vi "State Machine from Enum.vi"(6 "Variant in":variant, 7 "Shift Pressed?":bool, 8 "error in (no error)":errorcluster, 10 "QD Combo Box Ref":refnum<vi>, 11 "QD Launch VI Ref":refnum<vi>) -> (0 "error out":errorcluster, 4 "Variant out":variant)   [LabVIEW 2012, in "State Machine From Enum.lvlib"]
doc: "Goal :\n\nPretty much everyone uses state machines as this is a rather basic but efficient design pattern that can be mixed together with others DPs. Whichever the platform (RT, FPGA, Win), an application will most likely include a state machine (or more!).\n\nFirst thing : create the enum that will describe the states of the machine. Yeah well, with this QDKS, that's roughly the only thing you will need to do.\n\nHow-To :\n\n- Copy the attached QD VI to the usual directory.\n\n- Configure its key (S is fine !)\n\n- Select an enum terminal or constant in your BD. Make sure there is some free space at the right of the enum.\n\n- Ctrl+Space Ctrl+Key. You've earned a state machine corresponding to the enum items.\n\nDefault Shortcut - [S]"
uses:
  State Machine From Enum.lvlib
  <vilib>/Utility/miscctls.llb/LVPointTypeDef.ctl
  <vilib>/Utility/miscctls.llb/LVBoundsTypeDef.ctl
  <vilib>/Utility/miscctls.llb/LVPositionTypeDef.ctl
panel:
  in  "Undo Name":string="Quick Drop Keyboard Shortcut"
  # "Do not change the connector pane of this VI.\n\nSee the block diagram for directions on how to use this template."
  # "Specify the name of the Undo transaction"
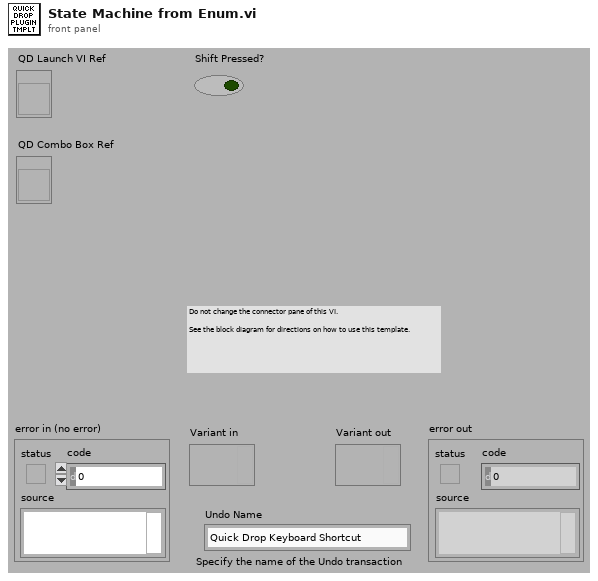
[diagram p1: front panel]
types:
  T1 = typedef "LVPositionTypeDef.ctl" = cluster{"Left":i32, "Top":i32}
  T2 = typedef "LVBoundsTypeDef.ctl" = cluster{"Width":u32, "Height":u32}
  T3 = typedef "LVPointTypeDef.ctl" = cluster{"Horizontal":i16, "Vertical":i16}
  T4 = enum32{"not a typedef", "typedef", "strict typedef", "class private data"}
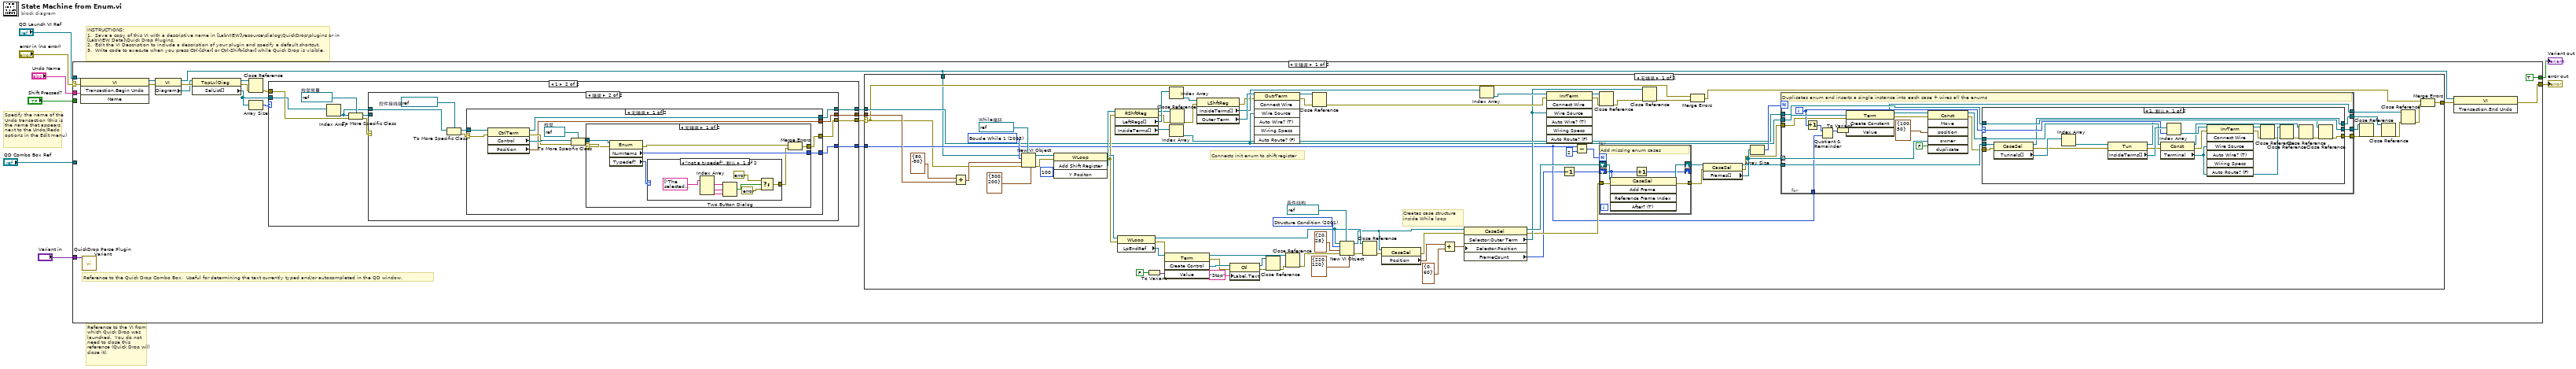
[diagram p0: block diagram]
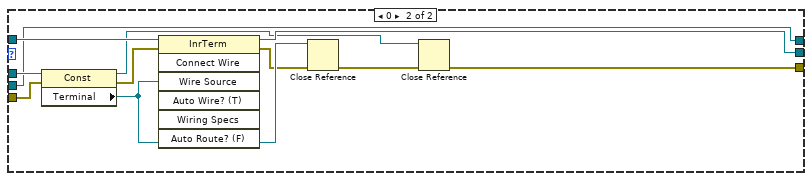
[diagram p2: hidden frame]
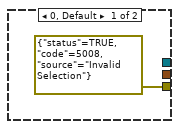
[diagram p4: hidden frame]
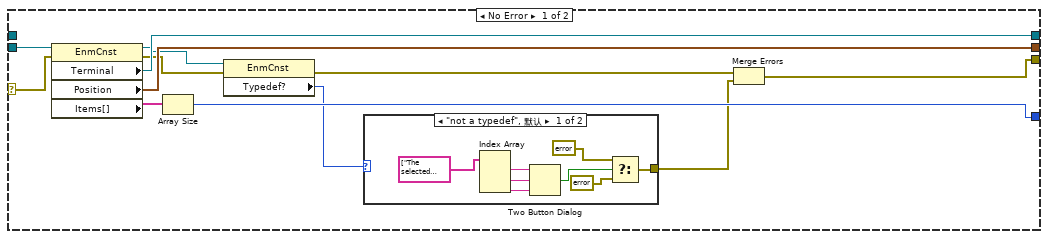
[diagram p5: hidden frame]
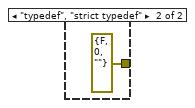
[diagram p6: hidden frame]
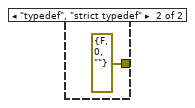
[diagram p7: hidden frame]
diagram:
  # "Specify the name of the Undo transaction (this is the name that appears next to the Undo/Redo options in the Edit menu)"
  # "Reference to the VI from which Quick Drop was launched.  You do not need to close this reference (Quick Drop will close it)."
  # "INSTRUCTIONS:\n1.  Save a copy of this VI with a descriptive name in [LabVIEW]\\resource\\dialog\\QuickDrop\\plugins or in [LabVIEW Data]\\Quick Drop Plugins.\n2.  Edit the VI Description to include a description of your plugin and specify a default shortcut. \n3.  Write code to execute when you press Ctrl-[char] or Ctrl-Shift-[char] while Quick Drop is visible."
  n1 = case shown="无错误" "error in (no error)" {
    selector: "error in (no error)" -> [w28 w239]
    tunnel: [w23 w239] -> w7
    tunnel: "QD Launch VI Ref" -> [w27 _]
    tunnel: "Shift Pressed?" -> [_ _]
    tunnel: "QD Combo Box Ref" -> [_ _]
    tunnel: "Variant in" -> [w29 _]
    tunnel: "Undo Name" -> [w26 _]
    tunnel: [TRUE _] -> w1
    frame No Error {
      # "Reference to the Quick Drop Combo Box.  Useful for determining the text currently typed and/or autocompleted in the QD window."
      n2 = invoke class="VI" method="Transaction.Begin Undo"(reference=w27, error in=w28, "Name"=w26) -> (reference out=w22:refnum<vi>, error out=w24:errorcluster)  [unwired: 1 in, 2 out]
      n3 = call <vilib>:"QuickDrop Parse Plugin Variant.vi"("QDKS Variant in"=w29) -> ()  [unwired: 12 in, 3 out]
      n4 = property class="VI"(reference=w22, error in=w24) -> (reference out=w9:refnum<vi>, error out=w17:errorcluster, "Diagram"=w16:refnum<vi>)
      n5 = property class="TopLvlDiag"(reference=w16, error in=w17) -> (reference out=w14:refnum<vi>, error out=w15:errorcluster, "SelList[]"=w20:refnum<vi>[])
      n6 = Close Reference(reference=w14, error in (no error)=w15) -> (error out=w19:errorcluster)
      n7 = Array Size(array=w20) -> (size(s)=w21:i32)
      n8 = case shown="1" w21 {
        tunnel: w20 -> [_ w180]
        tunnel: w19 -> [_ w179]
        tunnel: [errorcluster {"status"=TRUE, "code"=5008, "source"="Invalid Selection"} ("error IO") w178] -> w18
        tunnel: [_ w174] -> w12
        tunnel: [_ w173] -> w11
        tunnel: [_ w172] -> w10
        frame 0, Default {
        }
        frame 1 {
          w176 = refnum<vi> refnum  # 枚举常量
          n9 = Index Array(array=w180) -> (element=w171:refnum<vi>)  [unwired: 1 in]
          n10 = To More Specific Class(target class=w176, reference=w171, error in=w179) -> (specific class reference=w177:refnum<vi>, error out=w175:errorcluster)
          n11 = case shown="错误" w175 {
            selector: w175 -> [w190 _]
            tunnel: [w183 w206] -> w178
            tunnel: w177 -> [w191 _]
            tunnel: [w189 w205] -> w172
            tunnel: [w188 w204] -> w174
            tunnel: [w187 w203] -> w173
            tunnel: w171 -> [_ w202]
            frame No Error {
              n12 = property class="EnmCnst"(reference=w191, error in=w190) -> (reference out=w186:refnum<vi>, error out=w184:errorcluster, "Terminal"=w189:refnum<vi>, "Position"=w188:T1, "Items[]"=w192:string[])
              n13 = Array Size(array=w192) -> (size(s)=w187:i32)
              n14 = property class="EnmCnst"(reference=w186, error in=w184) -> (error out=w181:errorcluster, "Typedef?"=w185:T4)  [unwired: 1 out]
              n15 = case shown="\"not a typedef\", 默认" w185 {
                tunnel: [w193 errorcluster {"status"=FALSE, "code"=0, "source"=""} ("error IO")] -> w182
                frame "not a typedef", Default {
                  n16 = Index Array(array=string[] ["The selected enum is not a typedef (and you may not create a non-typedef'ed state machine !). \n\nDo you want to continue ?", "Yes", "No"]) -> (element #1=w199:string, element #2=w198:string, element #3=w197:string)  [unwired: 3 in]
                  n17 = Two Button Dialog(message=w199, 1:w197, 2:w198) -> (T button?=w196:bool)
                  n18 = Select(t=errorcluster {"status"=FALSE, "code"=0, "source"=" "} ("error IO"), s=w196, f=errorcluster {"status"=TRUE, "code"=5008, "source"="Invalid Selection"} ("error IO")) -> (s? t:f=w193:errorcluster)
                }
                frame "typedef", "strict typedef" {
                }
              }
              n19 = Merge Errors(w181, w182) -> (w183:errorcluster)
            }
            frame Error {
              w208 = refnum<vi> refnum  # 控件接线端
              n20 = To More Specific Class(target class=w208, reference=w202) -> (specific class reference=w209:refnum<vi>, error out=w207:errorcluster)  [unwired: 1 in]
              n21 = case shown="无错误" w207 {
                selector: w207 -> [w214 w238]
                tunnel: w209 -> [w220 _]
                tunnel: [w213 w238] -> w206
                tunnel: [w212 _] -> w205
                tunnel: [w211 _] -> w204
                tunnel: [w210 _] -> w203
                frame No Error {
                  w217 = refnum<vi> refnum  # 枚举
                  n22 = property class="CtrlTerm"(reference=w220, error in=w214) -> (reference out=w212:refnum<vi>, error out=w218:errorcluster, "Control"=w219:refnum<vi>, "Position"=w211:T1)
                  n23 = To More Specific Class(target class=w217, reference=w219, error in=w218) -> (specific class reference=w216:refnum<vi>, error out=w215:errorcluster)
                  n24 = case shown="无错误" w215 {
                    selector: w215 -> [w226 w237]
                    tunnel: w216 -> [w227 _]
                    tunnel: [w221 w237] -> w213
                    tunnel: [w225 _] -> w210
                    frame No Error {
                      n25 = property class="Enum"(reference=w227, error in=w226) -> (error out=w222:errorcluster, "NumItems"=w225:u32, "Typedef?"=w224:T4)  [unwired: 1 out]
                      n26 = case shown="\"not a typedef\", 默认" w224 {
                        tunnel: [w228 errorcluster {"status"=FALSE, "code"=0, "source"=""} ("error IO")] -> w223
                        frame "not a typedef", Default {
                          n27 = Index Array(array=string[] ["The selected enum is not a typedef (and you may not create a non-typedef'ed state machine !). \n\nDo you want to continue ?", "Yes", "No"]) -> (element #1=w234:string, element #2=w233:string, element #3=w232:string)  [unwired: 3 in]
                          n28 = Two Button Dialog(message=w234, 1:w232, 2:w233) -> (T button?=w231:bool)
                          n29 = Select(t=errorcluster {"status"=FALSE, "code"=0, "source"=" "} ("error IO"), s=w231, f=errorcluster {"status"=TRUE, "code"=5008, "source"="Invalid Selection"} ("error IO")) -> (s? t:f=w228:errorcluster)
                        }
                        frame "typedef", "strict typedef" {
                        }
                      }
                      n30 = Merge Errors(w222, w223) -> (w221:errorcluster)
                    }
                    frame Error {
                    }
                  }
                }
                frame Error {
                }
              }
            }
          }
        }
      }
      n31 = case shown="无错误" w18 {
        selector: w18 -> [w46 w169]
        tunnel: [w44 w169] -> w13
        tunnel: w12 -> [w49 _]
        tunnel: w11 -> [w48 _]
        tunnel: w10 -> [w47 _]
        tunnel: w9 -> [w45 _]
        frame No Error {
          w98 = refnum<vi> refnum  # 条件结构
          w99 = 2001 items=[" Additionner (avec terminaux d'erreur)"=3915, " Arbre (classique)"=21819, " Arbre (moderne)"=21793, " Arbre (système)"=21794, " Barre de défil. horiz. de dlg"=21905, " Barre de défil. vert. de dlg"=21906, " Barre de progression horizontale (moderne)"=21102, " Barre de progression horizontale (système)"=21910, " Barre de progression verticale (moderne)"=21104, " Barre de progression verticale (système)"=21909, " Bin 1"=3073, " Bin 2"=21755, " Boucle While 1"=2003, " Boucle While 2"=2352, " Bouton Annuler (moderne)"=21739, " Bouton Annuler (système)"=3131, " Bouton OK (moderne)"=21738, " Bouton OK (système)"=3130, " Bouton radio (système)"=3133, " Bouton rotatif (classique)"=3005, " Bouton rotatif (moderne)"=21000, " Bouton-poussoir carré"=3119, " Bouton-poussoir carré (profil)"=3113, " Bouton-poussoir circulaire"=3118, " Bouton-poussoir circulaire (profil)"=3112, " Boutons radio (classique)"=22003, " Boutons radio (moderne)"=22001, " Boutons radio (système)"=22002, " Boîte de couleur encadrée (classique)"=3008, " Boîte de couleur encadrée (moderne)"=21019, " Boîte de dialogue de fichier (obsolète)"=8081, " Boîte en relief (classique)"=3600, " Boîte en relief (moderne)"=3637, " Boîte épaisse (encastrée)"=3635, " Cadran (classique)"=3050, " Cadran (moderne)"=21732, " Cadre encastré (moderne)"=3607, " Cadre encastré (système)"=3624, " Case à cocher (classique)"=3117, " Case à cocher (moderne)"=21924, " Case à cocher (système)"=3132, " Case à cocher mixte (système)"=21333, " Chaîne de dlg"=2110, " Chaîne déroulante (classique)"=3304, " Chaîne déroulante (moderne)"=21604, " Chaîne déroulante (système)"=21917, " Cluster (classique)"=3400, " Cluster (moderne)"=21607, " Commande chaîne (classique)"=3200, " Commande chaîne (moderne)"=21701, " Commande chaîne (système)"=21920, " Commande chemin (classique)"=3203, " Commande chemin (moderne)"=21730, " Commande chemin (système)"=21922, " Commande horodatage (classique)"=5555, " Commande horodatage (moderne)"=21913, " Commande horodatage (système)"=21967, " Commande numérique (classique)"=3000, " Commande numérique (moderne)"=21003, " Commande numérique (système)"=21919, " Commande numérique à incrémentation (système)"=21900, " Commande onglets (classique)"=3330, " Commande onglets (moderne)"=3332, " Commande onglets (système)"=3331, " Commande variable partagée (classique)"=3472, " Commande variable partagée (moderne)"=21814, " Copier (obsolète)"=1416, " Coude gauche vers le bas (ombré)"=3711, " Coude gauche vers le bas (plat)"=3811, " Coude gauche vers le haut (ombré)"=3708, " Coude gauche vers le haut (plat)"=3808, " Coude vers le bas à droite (ombré)"=3717, " Coude vers le bas à droite (plat)"=3817, " Coude vers le haut à droite (ombré)"=3714, " Coude vers le haut à droite (plat)"=3814, " Diviser (avec terminaux d'erreur)"=3918, " Données numériques (classique)"=3210, " Données numériques (moderne)"=21216, " Déplacer (obsolète)"=1415, " Entonnoir 1"=21754, " Entonnoir 2"=3072, " Fermer un fichier (obsolète)"=1405, " Glissière horizontale (classique)"=3010, " Glissière horizontale (système)"=21904, " Glissière verticale (système)"=21903, " Glissière à curseur horizontale (classique)"=3011, " Glissière à curseur horizontale (moderne)"=21101, " Glissière à curseur horizontale (système)"=21902, " Glissière à curseur verticale (classique)"=3007, " Glissière à curseur verticale (moderne)"=21017, " Glissière à curseur verticale (système)"=21901, " Glissière à niveau horizontale (classique)"=3012, " Glissière à niveau horizontale (moderne)"=21100, " Glissière à niveau verticale (classique)"=3009, " Glissière à niveau verticale (moderne)"=21014, " Graphe (classique)"=3504, " Graphe (moderne)"=21703, " Graphe d'intensité (classique)"=3510, " Graphe d'intensité (moderne)"=21720, " Graphe déroulant (moderne)"=21717, " Graphe déroulant d'intensité (classique)"=3509, " Graphe déroulant d'intensité (moderne)"=21719, " Graphe numérique (classique)"=3511, " Graphe numérique (moderne)"=21718, " Graphe XY (classique)"=3500, " Graphe XY (moderne)"=21716, " Horodatage (constante du diagramme)"=2068, " Indicateur chaîne (classique)"=3201, " Indicateur chaîne (moderne)"=21702, " Indicateur chemin (classique)"=3204, " Indicateur chemin (moderne)"=21731, " Indicateur horodatage (classique)"=5556, " Indicateur horodatage (moderne)"=21914, " Indicateur numérique (classique)"=3001, " Indicateur numérique (moderne)"=21004, " Infos sur le fichier/répertoire (obsolète)"=1413, " Interface CAN (classique)"=3339, " Interface CAN (constante du diagramme)"=2123, " Interface CAN (moderne)"=21815, " Interface CAN (système)"=21964, " Interrupteur à bascule horizontal (classique)"=3110, " Interrupteur à bascule horizontal (moderne)"=21700, " Interrupteur à bascule vertical (classique)"=3111, " Interrupteur à bascule vertical (moderne)"=21005, " Interrupteur à glissière vertical (classique)"=3115, " Interrupteur à glissière vertical (moderne)"=21741, " Jauge (classique)"=3040, " Jauge (moderne)"=21009, " LED carrée (classique)"=3121, " LED carrée (moderne)"=21013, " LED circulaire (classique)"=3120, " LED circulaire (moderne)"=21012, " Ligne (ciselée, fine)"=3627, " Ligne (ciselée, système)"=3632, " Ligne (ciselée, épaisse)"=3630, " Ligne (fine)"=3626, " Ligne (épaisse)"=3629, " Ligne avec flèche (fine)"=3628, " Ligne avec flèche (épaisse)"=3631, " Liste déroulante (classique)"=21806, " Liste déroulante (moderne)"=21792, " Liste déroulante (système)"=21805, " Liste multicolonne (classique)"=21799, " Liste multicolonne (moderne)"=21791, " Liste multicolonne (système)"=21798, " Menu déroulant (classique)"=3018, " Menu déroulant (moderne)"=21600, " Menu déroulant d'images (classique)"=3015, " Menu déroulant d'images (moderne)"=21602, " Menu déroulant d'images (système)"=21925, " Menu déroulant texte (classique)"=3014, " Menu déroulant texte (constante du diagramme)"=2008, " Menu déroulant texte (moderne)"=21601, " Menu déroulant texte (système)"=3060, " Menu déroulant texte et images (classique)"=3016, " Menu déroulant texte et images (moderne)"=21603, " Mettre à jour le fichier (obsolète)"=1406, " Moteur (ombré)"=3720, " Moteur (plat)"=3820, " Multiplier (avec terminaux d'erreur)"=3917, " Nom d'échelle DAQmx (classique)"=3317, " Nom d'échelle DAQmx (constante du diagramme)"=2116, " Nom d'échelle DAQmx (moderne)"=21775, " Nom d'échelle DAQmx (système)"=21952, " Nom de périphérique DAQmx (classique)"=3318, " Nom de périphérique DAQmx (constante du diagramme)"=2093, " Nom de périphérique DAQmx (moderne)"=21773, " Nom de périphérique DAQmx (système)"=21950, " Nom de ressource VISA (classique)"=3409, " Nom de ressource VISA (moderne)"=21737, " Nom de tâche DAQmx (classique)"=3442, " Nom de tâche DAQmx (constante du diagramme)"=3434, " Nom de tâche DAQmx (moderne)"=21778, " Nom de tâche DAQmx (système)"=21959, " Nom logique IVI (classique)"=3414, " Nom logique IVI (constante du diagramme)"=3420, " Nom logique IVI (moderne)"=21736, " Numérique de dlg 1"=2100, " Numérique de dlg 2"=3006, " Pixmap (attention : dangereux)"=3507, " Point d'E/S FieldPoint (classique)"=3439, " Point d'E/S FieldPoint (constante du diagramme)"=3440, " Point d'E/S FieldPoint (moderne)"=21784, " Pompe vers la droite (ombrée)"=3719, " Pompe vers la droite (plate)"=3819, " Pompe vers la gauche (ombrée)"=3713, " Pompe vers la gauche (plate)"=3813, " RecomposerRéfValDonnéesDéverrou (warning: dangerous)"=2407, " RecomposerVariant (warning: dangerous)"=2405, " Rectangle de couleur (brisé ?)"=3625, " Ressource Motion (classique)"=3448, " Ressource Motion (constante du diagramme)"=3449, " Ressource Motion (moderne)"=21787, " Réservoir (classique)"=3020, " Réservoir (moderne)"=21006, " Réservoir atmosphérique (classique)"=3070, " Réservoir atmosphérique (moderne)"=21751, " Réservoir de pression (ombré)"=21753, " Réservoir de pression (plat)"=3075, " Réservoir ouvert (ombré classique)"=3074, " Réservoir ouvert (plat classique)"=21752, " Soupape courbée vers la droite (contour)"=3805, " Soupape courbée vers la droite (ombrée)"=21765, " Soupape courbée vers la droite (plate)"=3705, " Soupape courbée vers la gauche (contour)"=3801, " Soupape courbée vers la gauche (ombrée)"=21761, " Soupape courbée vers la gauche (plate)"=3701, " Soupape courbée vers le bas (contour)"=3807, " Soupape courbée vers le bas (ombrée)"=21767, " Soupape courbée vers le bas (plate)"=3707, " Soupape courbée vers le haut (contour)"=3803, " Soupape courbée vers le haut (ombrée)"=21763, " Soupape courbée vers le haut (plate)"=3703, " Soupape rectangulaire vers la droite (contour)"=3804, " Soupape rectangulaire vers la droite (ombrée)"=21764, " Soupape rectangulaire vers la droite (plate)"=3704, " Soupape rectangulaire vers la gauche (contour)"=3800, " Soupape rectangulaire vers la gauche (ombrée)"=21760, " Soupape rectangulaire vers la gauche (plate)"=3700, " Soupape rectangulaire vers le bas (contour)"=3806, " Soupape rectangulaire vers le bas (ombrée)"=21766, " Soupape rectangulaire vers le bas (plate)"=3706, " Soupape rectangulaire vers le haut (contour)"=21762, " Soupape rectangulaire vers le haut (ombrée)"=3802, " Soupape rectangulaire vers le haut (plate)"=3702, " Source de déclenchement analogique DAQmx (classique)"=3336, " Source de déclenchement analogique DAQmx (constante du diagramme)"=2119, " Source de déclenchement analogique DAQmx (moderne)"=21774, " Source de déclenchement analogique DAQmx (système)"=21951, " Soustraire (avec terminaux d'erreur)"=3916, " Supprimer (obsolète)"=1417, " Switch DAQmx (classique)"=3337, " Switch DAQmx (constante du diagramme)"=2121, " Switch DAQmx (moderne)"=21776, " Switch DAQmx (système)"=21953, " Table (classique)"=21796, " Table (moderne)"=21790, " Table (système)"=21797, " Tableau (classique)"=3300, " Tableau (constante du diagramme)"=2070, " Tableau (moderne)"=21608, " Tag de refnum défini par l'utilisateur (classique)"=3429, " Tag de refnum défini par l'utilisateur (constante du diagramme)"=3426, " Tag de refnum défini par l'utilisateur (moderne)"=21745, " Tag de refnum défini par l'utilisateur aplati (classique)"=3454, " Tag de refnum défini par l'utilisateur aplati (modern)"=21747, " Tag défini par l'utilisateur aplati (moderne)"=21749, " Tag défini par utilisateur (classique)"=3329, " Tag défini par utilisateur (constante du diagramme)"=2114, " Tee vers la droite (ombré)"=3715, " Tee vers la droite (plat)"=3815, " Tee vers la gauche (ombré)"=3709, " Tee vers la gauche (plat)"=3809, " Tee vers le bas (ombré)"=3718, " Tee vers le bas (plat)"=3818, " Tee vers le haut (ombré)"=3712, " Tee vers le haut (plat)"=3812, " Terminal DAQmx (classique)"=3319, " Terminal DAQmx (constante du diagramme)"=2117, " Terminal DAQmx (moderne)"=21781, " Terminal DAQmx (système)"=21955, " Thermomètre (classique)"=3021, " Thermomètre (moderne)"=21007, " Tuyau horiz. (ombré)"=3710, " Tuyau horiz. (plat)"=3810, " Tuyau vertical (ombré)"=3716, " Tuyau vertical (plat)"=3816, " Tâche CAN (classique)"=3470, " Tâche CAN (constante du diagramme)"=3471, " Tâche CAN (moderne)"=21789, " Tâche CAN (système)"=21963, " Voie CAN (classique)"=3340, " Voie CAN (constante du diagramme)"=2124, " Voie CAN (moderne)"=21817, " Voie CAN (système)"=21966, " Voie de NI-DAQ traditionnel (classique)"=3320, " Voie de NI-DAQ traditionnel (constante du diagramme)"=2085, " Voie de NI-DAQ traditionnel (moderne)"=21733, " Voie globale DAQmx (classique)"=3443, " Voie globale DAQmx (constante du diagramme)"=3430, " Voie globale DAQmx (moderne)"=21770, " Voie globale DAQmx (système)"=21957, " Voie physique DAQmx (classique)"=3335, " Voie physique DAQmx (constante du diagramme)"=2118, " Voie physique DAQmx (moderne)"=21777, " Voie physique DAQmx (système)"=21954, " Vumètre (classique)"=3030, " Vumètre (moderne)"=21008, " Écrire dans un fichier binaire"=8078, " Écrire dans un fichier texte"=8080, " Énum (classique)"=3023, " Énum (moderne)"=21605, " Énum (système)"=3062, " Étiquette (moderne)"=21960, " Étiquette (système)"=21961, "Activer le repérage des menus"=9002, "Adapter d'entier à virgule fixe"=5567, "Adapter de virgule fixe à entier"=5566, "Adapter le type"=1166, "Additionner"=1050, "Additionner les éléments du tableau"=1903, "Agitateur"=3831, "Ajouter la chaîne Vrai/Faux"=1511, "Ajouter un élément au début d'une file d'attente"=9129, "Ajouter un élément à la fin d'une file d'attente"=9111, "Ajouter un élément à la fin d'une file d'attente avec pertes"=9130, "Ajouter une chaîne multiligne"=1510, "AllSpoll"=1960, "Ampoule carrée"=3105, "Ampoule circulaire"=3104, "Ancien VISA Open"=1921, "Annuler une notification"=9107, "Aperçu du premier élément d'une file d'attente"=9112, "Aplatir en chaîne"=1164, "Aplatir en XML"=8400, "Appel par référence MathScript"=3906, "Appeler la méthode parente"=2354, "Appeler par référence"=3901, "Appeler une fonction d'une DLL"=2062, "Arc cosinus"=1207, "Arc cosinus hyperbolique"=1218, "Arc cosécante"=23050, "Arc cosécante hyperbolique"=23056, "Arc cotangente"=23052, "Arc cotangente hyperbolique"=23058, "Arc sinus"=1206, "Arc sinus hyperbolique"=1217, "Arc sécante"=23051, "Arc sécante hyperbolique"=23057, "Arc tangente"=1208, "Arc tangente (2 entrées)"=1228, "Arc tangente hyperbolique"=1219, "Array Interface Control"=23777, "Arrondir vers +l'infini"=1076, "Arrondir vers -l'infini"=1075, "Arrondir à l'entier le plus proche"=1055, "Arrêter"=1350, "Assembler"=2049, "Assembler des signaux"=2350, "Assembler par nom"=2057, "Attendre (ms)"=1302, "Attendre un multiple de ms"=1327, "Attendre une activité sur la face-avant"=1328, "Attendre une notification"=9105, "Attendre une notification avec historique des notificateurs"=9131, "Attendre une notification de plusieurs"=9106, "Attendre une notification de plusieurs avec historique des notificateurs"=9132, "Attendre une occurrence"=1701, "Attente d'activité"=1722, "Automation Fermer"=8001, "Automation Ouvrir"=8000, "Balayer un fichier"=2082, "Balayer une chaîne"=2080, "Balayer une valeur"=1534, "Barre de division horizontale"=21861, "Barre de division horizontale (classique)"=21863, "Barre de division horizontale (système)"=21865, "Barre de division verticale"=21860, "Barre de division verticale (classique)"=21862, "Barre de division verticale (système)"=21864, "Barre de défilement horizontale"=21110, "Barre de défilement verticale"=21111, "Barre de menus du VI actuel"=9000, "Barre graduée horizontale"=21106, "Barre graduée verticale"=21107, "Base du logarithme népérien"=23510, "Bibliothèque de VIs"=1425, "Bitpack en tableau"=3135, "Bluetooth - Attendre un récepteur"=9147, "Bluetooth - Créer un récepteur"=9151, "Bluetooth - Découvrir"=9152, "Bluetooth - Fermer la connexion"=9148, "Bluetooth - Lire"=9149, "Bluetooth - Ouvrir une connexion"=9153, "Bluetooth - Écrire"=9150, "Booléen en (0,1)"=1167, "Boucle cadencée"=5570, "Boucle de contrôle et simulation"=2099, "Boucle For"=2002, "Bouton allongé à étiquette"=3125, "Bouton carré"=3101, "Bouton carré plat"=3103, "Bouton carré plat de plate-forme"=3134, "Bouton carré à étiquette"=3123, "Bouton circulaire"=3100, "Bouton circulaire à étiquette"=3122, "Bouton LED"=3116, "Bouton radio carré"=3107, "Bouton radio circulaire"=3106, "Bouton rectangulaire à étiquette"=3124, "Bouton rond plat"=3102, "Bouton Stop"=21230, "Bouton Stop circulaire"=3127, "Bouton Stop rectangulaire"=3128, "Bouton Texte"=21015, "Bouton-poussoir"=21001, "Boîte arrondie en relief"=3609, "Boîte arrondie encastrée"=3638, "Boîte arrondie encastrée 1"=3610, "Boîte arrondie plate"=3611, "Boîte bouton horizontale"=3636, "Boîte de calcul"=2004, "Boîte de couleur"=3013, "Boîte de couleur à bord mince"=2905, "Boîte de dialogue de fichier"=8058, "Boîte de dialogue à deux boutons"=1341, "Boîte de dialogue à un bouton"=1340, "Boîte encastrée"=3601, "Boîte lisse horizontale"=3633, "Boîte lisse verticale"=3634, "Boîte plate"=3602, "Cadre en relief"=3606, "Cadre plat"=3608, "Carré"=23059, "Casting dynamique d'interface FPGA"=5690, "Cercle en relief"=3603, "Cercle encastré"=3604, "Cercle plat"=3605, "Changer les bases d'unités"=1079, "Charge élémentaire (C)"=23517, "Chaîne aplatie en variant"=8202, "Chaîne au format tableur en tableau"=1539, "Chaîne d'appel"=1999, "Chaîne de date/heure"=1600, "Chaîne décimale en nombre"=1184, "Chaîne en chemin"=1078, "Chaîne en IP"=1711, "Chaîne en tableau d'octets"=1608, "Chaîne en variable partagée"=1830, "Chaîne Fract/Exp en nombre"=1187, "Chaîne hexadécimale en nombre"=1185, "Chaîne octale en nombre"=1186, "Chaîne simple"=2115, "Chemin du VI actuel"=1426, "Chemin en chaîne"=1077, "Chemin en tableau de chaînes"=1423, "Chemin/Chaîne vide ?"=1112, "Chiffre décimal ?"=1119, "Chiffre hexa ?"=1123, "Chiffre octal ?"=1129, "Classe lexicale"=1126, "Classer un tableau 1D"=1120, "Cluster en tableau"=1169, "Code Interface Node"=2050, "Commande Plug-In"=21820, "Commande/état du périphérique"=1433, "Complexe conjugué"=1048, "Complexe en polaire"=1045, "Complexe en Réel/Im"=1044, "Composer un chemin"=1419, "Compresseur"=3832, "Compteur d'impulsions d'horloge (ms)"=1300, "Concaténer des chaînes"=2040, "Constante 'Pas un chemin'"=23524, "Constante 'Pas un refnum'"=23526, "Constante boîte de couleur"=2120, "Constante chaîne"=2007, "Constante chaîne déroulante"=2088, "Constante chaîne vide"=23503, "Constante chemin"=2009, "Constante chemin vide"=23523, "Constante cluster"=2071, "Constante d'Avogadro (1/mol)"=23520, "Constante de Planck (J/Hz)"=23516, "Constante de Rydberg (1/m)"=23521, "Constante de spécification de classe"=2094, "Constante de spécification de classe de variable"=2106, "Constante des gaz parfaits (J/(mol K))"=23522, "Constante Faux"=2006, "Constante fin de ligne"=23525, "Constante gravitationnelle"=23519, "Constante menu déroulant d'erreurs"=2039, "Constante menu déroulant de symboles"=2038, "Constante Nom de variable"=3478, "Constante numérique"=2005, "Constante Retour chariot"=23500, "Constante Retour à la ligne"=23501, "Constante référence de valeur de données"=24134, "Constante tabulation"=23502, "Constante variable partagée"=3473, "Constante énumération"=2090, "Construire un tableau"=2041, "Construire un tableau de clusters"=2047, "Construire une matrice"=8500, "Construire une waveform"=2066, "Conteneur .NET"=2125, "Conteneur ActiveX"=2072, "Contraindre au type"=2402, "Contrôle de l'aide en ligne"=1355, "Contrôle de la fenêtre d'aide"=1353, "Convertir une unité"=2059, "Copier"=8053, "Correspondance de chaîne Vrai/Faux"=1533, "Cosinus"=1201, "Cosinus hyperbolique"=1215, "Cosécante"=1204, "Cosécante hyperbolique"=23053, "Cotangente"=1205, "Cotangente hyperbolique"=23055, "Créer l'extrémité d'écriture d'un flux réseau"=23810, "Créer l'extrémité de lecture d'un flux réseau"=23811, "Créer un dossier"=8055, "Créer un flux"=23796, "Créer un événement utilisateur"=2073, "Créer une FIFO RT"=24000, "Culbuteur"=21002, "Culbuteur vertical"=21740, "Dans la gamme"=1127, "DataSocket Fermer"=1085, "DataSocket Lire"=1086, "DataSocket Ouvrir"=1084, "DataSocket Écrire"=1087, "Date et heure en secondes"=1303, "Date/heure en secondes"=1308, "Demander une désallocation"=1610, "DevClear"=1961, "DevClearList"=1962, "Diagramme d'états"=2051, "Diffuser la référence de valeur Variant"=2410, "Différent de 0 ?"=1116, "Différents ?"=1105, "Dimensionner le handle"=1603, "Distributeur rotatif"=3830, "Diviser"=1053, "Diviser un tableau 1D"=1908, "Droits d'accès"=1412, "Décalage logique"=1081, "Décimer un tableau 1D"=2046, "Décomposer un chemin"=1420, "DécomposerRéfValDonnéesVerrou"=2406, "DécomposerTableau"=2412, "DécomposerVariant"=2404, "Découper un nombre"=1170, "Décrémenter"=1058, "Défaire un package de matrice"=23000, "Définir des éléments de matrice"=8505, "Définir la position dans le fichier"=8073, "Définir la position dans le fichier journal LabVIEW"=8072, "Définir la taille du fichier"=8074, "Définir le nombre d'enregistrements"=8075, "Définir le type et le créateur"=8077, "Définir les autorisations"=8076, "Définir les infos de l'élément de menu"=9006, "Définir un attribut de variant"=8204, "Définir un attribut de waveform"=8207, "Définir une diagonale de matrice"=8504, "Définir une occurrence"=1702, "Définir une sous-matrice"=8506, "Dépassement des données à virgule fixe ?"=5565, "Déplacer"=8068, "Désassembler"=2048, "Désassembler des signaux"=2351, "Désassembler par nom"=2058, "Désenregistrement aux événements"=2076, "Détruire une extrémité d'un flux"=23794, "Effacer l'état de dépassement de virgule fixe"=5562, "En chaîne de sonde"=2413, "En complexe double précision"=1152, "En complexe précision étendue"=1154, "En complexe simple précision"=1151, "En entier de type octet"=1140, "En entier long"=1142, "En entier long non signé"=1145, "En entier mot"=1141, "En entier mot non signé"=1144, "En entier octet non signé"=1143, "En entier quad"=1155, "En entier quad non signé"=1156, "En flottant double précision"=1147, "En flottant précision étendue"=1149, "En flottant simple précision"=1146, "En horodatage"=5560, "En majuscules"=1188, "En minuscules"=1189, "En une classe plus générique"=8017, "En une classe plus spécifique"=8016, "En variant"=8201, "En variant OLE"=8002, "En virgule fixe"=5561, "EnableLocal"=1963, "EnableRemote"=1964, "Enregistrement à des événements"=2065, "Enregistrer un VI Callback d'événement"=2078, "Entrelacer des tableaux 1D"=2045, "Envoyer une notification"=9104, "EOF"=1410, "Epsilon machine"=23528, "Espace blanc ?"=1125, "ET"=1061, "ET logique entre les éléments du tableau"=1911, "Exponentielle"=1211, "Exponentielle (Arg) -1"=1222, "Face-avant secondaire"=21810, "Face-avant secondaire (classique)"=21811, "Face-avant secondaire (système)"=21823, "Faire un package de matrice"=23001, "Fermer un fichier"=8052, "Fermer une connexion à une variable"=23783, "Fermer une référence"=8011, "Fichier TDMS"=3477, "FindLstn"=1965, "FindRQS"=1966, "Flèche droite"=3825, "Flèche gauche"=3826, "Flèche vers le bas"=3824, "Flèche vers le haut"=3823, "Formater dans un fichier"=2083, "Formater en chaîne"=2081, "Formater la chaîne de date/heure"=8100, "Formater une valeur"=1512, "Four"=3829, "Fourche"=2194, "Fusionner les erreurs"=2147, "Glissière horizontale simple"=3003, "Glissière verticale"=3004, "Glissière verticale simple"=3002, "GPIB Clear"=1954, "GPIB Initialization"=1957, "GPIB Misc"=1956, "GPIB Read"=1951, "GPIB Serial Poll"=1955, "GPIB Status"=1959, "GPIB Trigger"=1953, "GPIB Wait"=1958, "GPIB Write"=1950, "Graphe de signaux mixte"=21721, "Graphe déroulant"=3501, "Graphe déroulant 1"=21010, "Générer un événement de suivi défini par l'utilisateur"=2250, "Générer un événement utilisateur"=2074, "Générer une activité sur la face-avant"=1329, "Générer une occurrence"=1700, "Handle Peek"=1604, "Handle Poke"=1605, "ID du processeur actuel"=24131, "Image 2D"=3508, "Image 3D"=23776, "Implique"=1080, "Imprimable ?"=1124, "Inclure l'état de dépassement de virgule fixe"=5564, "Incrémenter"=1057, "Indexer et assembler un tableau de clusters"=2056, "Indexer un tableau"=2042, "Indexer un tableau de chaînes"=1531, "Indice de ressource"=1088, "Informations sur le processeur"=24130, "Infos sur le fichier/répertoire"=8082, "Infos sur le volume"=1414, "Infos sur un raccourci de menu"=9007, "Infos sur un élément de menu"=9005, "Inférieur ?"=1111, "Inférieur ou égal ?"=1104, "Inférieur ou égal à 0 ?"=1115, "Inférieur à 0 ?"=1118, "Initialiser un tableau"=2053, "Inlining du nœud C"=2104, "Insérer dans un tableau"=3911, "Insérer des éléments de menu"=9003, "Interdire l'accès"=8057, "Interpoler un tableau 1D"=1905, "Interrupteur horizontal"=3108, "Interrupteur vertical"=3109, "Interrupteur à glissière"=21011, "Interrupteur à glissière horizontal"=3114, "Inverse de e"=23511, "Inverse de Pi"=23507, "Inverser"=1059, "Inverser un tableau 1D"=1900, "Inverser une chaîne"=1537, "IP en chaîne"=1710, "IrDA Attendre un récepteur"=9143, "IrDA Créer un récepteur"=9140, "IrDA Découvrir"=9141, "IrDA Fermer la connexion"=9144, "IrDA Lire"=9145, "IrDA Ouvrir une connexion"=9142, "IrDA Écrire"=9146, "Jauge pour Simon"=32600, "Joint"=2195, "Jonction"=2197, "Lecture directe de la variable "=23785, "Lecture par balayage de la variable"=23784, "Libérer un notificateur"=9102, "Libérer une file d'attente"=9109, "Ligne horiz."=3821, "Ligne verticale"=3822, "Lire plusieurs éléments du flux"=23803, "Lire un fichier"=1407, "Lire un fichier binaire"=8051, "Lire un fichier binaire avec préallocation"=24135, "Lire un fichier journal LabVIEW"=8069, "Lire un fichier texte"=8070, "Lire un périphérique"=1432, "Lire un seul élément du flux"=23797, "Lire une FIFO RT"=24001, "Lire une variable"=23781, "Lire une variable avec timeout"=23786, "Lister le contenu d'un répertoire"=1418, "Lister le contenu du dossier"=8083, "Logarithme base 10 de e"=23512, "Logarithme en base 10"=1210, "Logarithme en base 2"=1225, "Logarithme en base X"=1224, "Logarithme népérien"=1209, "Logarithme népérien (Arg +1)"=1221, "Logarithme népérien de 10"=23513, "Logarithme népérien de 2"=23514, "Logarithme népérien de Pi"=23508, "Longueur d'une chaîne"=1502, "MakeAddr"=1967, "Mantisse et exposant"=1150, "Max. et min."=1108, "Max. et min. d'un tableau"=1907, "Menu déroulant"=3061, "Menu déroulant d'attribut du tag"=2063, "Menu déroulant en retrait"=3019, "Menu déroulant popup"=3017, "Mettre à jour le fichier"=8059, "Moins l'infini"=23509, "Multiplier"=1052, "Multiplier les éléments du tableau"=1904, "Multiplier par une puissance de 2"=1074, "Ne pas diffuser la référence de valeur Variant"=2411, "Nom de ressource VISA"=3421, "Nombre aléatoire (0-1)"=1070, "Nombre de niveaux du cache"=24133, "Nombre en chaîne au format ingénieur"=1183, "Nombre en chaîne décimale"=1180, "Nombre en chaîne exponentielle"=1505, "Nombre en chaîne fractionnaire"=1506, "Nombre en chaîne hexadécimale"=1181, "Nombre en chaîne octale"=1182, "Nombre en tableau de booléens"=1814, "Non"=1064, "Non ET"=1071, "Non OU"=1072, "Non OU exclusif"=1073, "Nouveau fichier"=1404, "Nouveau répertoire"=1402, "Nouveau VI"=8014, "Nouvel objet de VI"=8015, "Nouvelle référence de valeur de données"=2408, "Nouvelle session IVI"=8102, "Numérique simple"=2900, "Nœud d'expression"=2201, "Nœud de données d'événement"=2102, "Nœud de méthode"=3900, "Nœud de propriété"=1920, "Nœud de rétroaction"=2353, "Nœud du constructeur"=3904, "Nœud MathScript"=2357, "Objet LabVIEW"=3457, "Obtenir des composantes à virgule fixe"=11163, "Obtenir l'état d'un notificateur"=9103, "Obtenir l'état d'une file d'attente"=9110, "Obtenir la diagonale d'une matrice"=8501, "Obtenir la position dans le fichier"=8062, "Obtenir la position dans le fichier journal LabVIEW"=8061, "Obtenir la taille du fichier"=8063, "Obtenir le nombre d'enregistrements"=8064, "Obtenir le type et le créateur"=8066, "Obtenir les autorisations"=8065, "Obtenir les composantes d'une waveform"=2067, "Obtenir les données glissées et déposées"=9154, "Obtenir les infos sur le volume"=8067, "Obtenir les éléments d'une matrice"=8502, "Obtenir un attribut de variant"=8205, "Obtenir un attribut de waveform"=8208, "Obtenir un notificateur"=9101, "Obtenir une file d'attente"=9108, "Obtenir une sous-matrice"=8503, "Opposé"=1069, "Opérateur arithmétique"=2200, "OU"=1062, "OU exclusif"=1063, "OU logique entre les éléments du tableau"=1910, "Ouvrir et vérifier la connexion d'une variable"=23790, "Ouvrir un fichier"=1403, "Ouvrir un périphérique"=1430, "Ouvrir une référence d'application"=8012, "Ouvrir une référence d'objet de VI"=8013, "Ouvrir une référence de VI"=8010, "Ouvrir/Créer/Remplacer un fichier"=8050, "Ouvrir/Créer/Remplacer un fichier journal LabVIEW"=8054, "Ovale lissé"=32500, "Ovale ombré"=32509, "Ovale à gradient horizontal"=32502, "Ovale à gradient vertical"=32501, "Partie de bouton"=21020, "Pas un nombre/chemin/refnum ?"=1128, "Pas une variable partagée"=23527, "PassControl"=1968, "Permuter les mots"=1163, "Permuter les octets"=1162, "Permuter les valeurs"=2401, "Permuter les éléments de vecteur"=1912, "Pi"=23504, "Pi / 2"=23506, "Pi x 2"=23505, "Pixmap"=3505, "Plus l'infini"=23515, "Polaire en complexe"=1047, "Polaire en Réel/Im"=23061, "PPoll"=1969, "PPollConfig"=1970, "PPollUnconfig"=1971, "Premier appel ?"=1083, "Préserver la classe à l'exécution"=8018, "Puissance de 10"=1212, "Puissance de 2"=1223, "Puissance de X"=1213, "Quitter LabVIEW"=1352, "Quotient et Reste"=1056, "Racine carrée"=1060, "Racine y-ième de x"=23062, "Rampe de couleur"=3022, "RcvRespMsg"=1972, "ReadStatus"=1973, "Receive"=1974, "ReceiveSetup"=1975, "Rechercher"=1409, "Rechercher dans un conteneur de variables"=23802, "Rechercher dans un tableau 1D"=1901, "Rechercher des symboles"=8101, "Rechercher et remplacer une chaîne"=3914, "Rechercher la première occurrence"=1532, "Rechercher une expression"=1535, "Rechercher/Découper une chaîne"=1538, "RecomperTableau"=2403, "Rectangle arrondi lissé"=32505, "Rectangle arrondi ombré"=32508, "Rectangle arrondi à gradient horizontal"=32507, "Rectangle arrondi à gradient vertical"=32506, "Rectangle à gradient horizontal"=32504, "Rectangle à gradient vertical"=32503, "Redimensionner un tableau"=2055, "Redimensionner une matrice"=8508, "Redresser à partir d'une chaîne"=1165, "Redresser à partir d'XML"=8401, "Refnum Automation"=3410, "Refnum d'application"=3412, "Refnum d'occurrence"=3406, "Refnum DataSocket"=3417, "Refnum de .NET"=3441, "Refnum de Callback d'événement"=3435, "Refnum de commande"=3419, "Refnum de connexion réseau Bluetooth"=3468, "Refnum de connexion réseau IrDA"=3450, "Refnum de connexion réseau TCP"=3407, "Refnum de connexion réseau UDP"=3418, "Refnum de fichier journal LabVIEW"=3402, "Refnum de fichier à flux d'octets"=3408, "Refnum de FIFO"=3474, "Refnum de file d'attente"=3424, "Refnum de menu"=3413, "RefNum de notificateur"=3423, "Refnum de périphérique"=3405, "Refnum de VI"=3422, "Refnum défini par l'utilisateur"=3428, "Refnum en chemin"=1424, "Refnum en session"=2306, "Refnum FPGA en session"=2322, "Regrouper des nombres"=1171, "Remplacer une portion d'un tableau"=3910, "Remplacer une portion de chaîne"=3913, "ResetSys"=1976, "Rotation"=1082, "Rotation dans un tableau 1D"=1906, "Rotation dans une chaîne"=1536, "Rotation droite avec retenue"=1607, "Rotation gauche avec retenue"=1606, "Réel/Im en complexe"=1046, "Réel/Im en polaire"=23060, "Référence de valeur de données"=3476, "Référence de VI Serveur"=2091, "Référence de VI statique"=2084, "Région"=2196, "Répertoire par défaut"=1427, "Répertoire temporaire"=1435, "Réservoir horizontal"=3071, "Script MATLAB"=9020, "Secondes en date/heure"=1309, "Send"=1977, "SendCmds"=1978, "SendDataBytes"=1979, "SendIFC"=1980, "SendList"=1981, "SendLLO"=1982, "SendSetup"=1983, "Session d'enregistrement"=2319, "Session en refnum"=2307, "Session IMAQ"=3415, "Session non enregistrée"=2320, "SetRWLS"=1984, "SetTimeOut"=1985, "Seuil d'un tableau 1D"=1909, "Signe"=1049, "Sinc"=1227, "Sinus"=1200, "Sinus et cosinus"=1220, "Sinus hyperbolique"=1214, "Sous-ensemble d'un tableau"=2044, "Sous-ensemble d'une chaîne"=1503, "Soustraire"=1051, "Structure Condition"=2001, "Structure multifréquence"=2199, "Structure Séquence déroulée"=2069, "Structure Séquence empilée"=2000, "Structure à conditions désactivées"=2064, "Structure à diagrammes désactivés"=2054, "Structure Élément en place"=2360, "Structure Événement"=2052, "Supprimer"=8056, "Supprimer des éléments de menu"=9004, "Supprimer l'état de dépassement de virgule fixe"=5563, "Supprimer la session IVI"=8103, "Supprimer le premier élément d'une file d'attente"=9113, "Supprimer un attribut de variant"=8206, "Supprimer un attribut de waveform"=8209, "Supprimer un événement utilisateur"=2075, "Supprimer une FIFO RT"=24003, "Supprimer une portion d'un tableau"=3912, "Supprimer une référence de valeur de données"=2409, "Supérieur ?"=1110, "Supérieur ou égal ?"=1103, "Supérieur ou égal à 0 ?"=1114, "Supérieur à 0 ?"=1117, "Sécante"=1203, "Sécante hyperbolique"=23054, "Sélectionner"=1516, "Séquence cadencée"=5573, "Tableau bitpack en données"=3136, "Tableau d'octets en chaîne"=1609, "Tableau de booléens en nombre"=1815, "Tableau de chaînes en chemin"=1422, "Tableau en chaîne au format tableur"=1540, "Tableau en cluster"=1168, "Tableau vide ?"=23063, "Taille d'un tableau"=1809, "Taille de matrice"=8507, "Taille du cache de données"=24132, "Tangente"=1202, "Tangente hyperbolique"=1216, "Tapis roulant"=3827, "TCP Attendre un récepteur"=1712, "TCP Créer un récepteur"=1717, "TCP Fermer la connexion"=1713, "TCP Lire"=1716, "TCP Lire des données Flex"=1720, "TCP Lire des données plates"=1718, "TCP Ouvrir une connexion"=1715, "TCP Écrire"=1714, "TCP Écrire des données Flex"=1721, "TCP Écrire des données plates"=1719, "TDMS - Configurer des lectures asynchrones (réf de données)"=2153, "TDMS - Configurer des écritures asynchrones (réf de données)"=2152, "TDMS - Lecture asynchrone (Avancée) (réf de données)"=2151, "TDMS - Obtenir l'état des lectures asynchrones (réf de données)"=2155, "TDMS - Obtenir l'état des écritures asynchrones (réf de données)"=2154, "TDMS - Écriture asynchrone (Avancée) (réf de données)"=2150, "TDMS Close"=24113, "TDMS Defragment"=24119, "TDMS Flush"=24117, "TDMS Get Properties"=24115, "TDMS List Contents"=24116, "TDMS Open"=24112, "TDMS Read"=24111, "TDMS Refnum To File ID"=24120, "TDMS Set Properties"=24114, "TDMS Write"=24110, "TDMS Write IP"=24118, "TestSRQ"=1986, "TestSys"=1987, "Texte en UTF-8"=23066, "Toujours copier"=2400, "Transposer un tableau 1D"=23068, "Transposer un tableau 2D"=1902, "Transposée d'une matrice"=8509, "Triangle en relief vers la droite"=3613, "Triangle en relief vers la gauche"=3612, "Triangle en relief vers le bas"=3615, "Triangle en relief vers le haut"=3614, "Triangle encastré vers la droite"=3617, "Triangle encastré vers la gauche"=3616, "Triangle encastré vers le bas"=3619, "Triangle encastré vers le haut"=3618, "Triangle plat vers la droite"=3621, "Triangle plat vers la gauche"=3620, "Triangle plat vers le bas"=3623, "Triangle plat vers le haut"=3622, "Trier un tableau de chaînes"=23065, "Trigger"=1988, "TriggerList"=1989, "Tuyau à plusieurs segments"=23780, "Type de chemin"=1421, "Type et créateur"=1434, "UDP Fermer"=1726, "UDP Lire"=1724, "UDP Multicast - Ouvrir"=1727, "UDP Ouvrir"=1723, "UDP Écrire"=1725, "UTF-8 en texte"=23067, "Valeur absolue"=1054, "Variable globale"=2060, "Variable locale"=2061, "Variable partagée"=23778, "Variable partagée en chaîne"=1831, "Variant"=3310, "Variant en chaîne aplatie"=8203, "Variant en donnée"=8003, "Variant OLE"=3150, "Verrouiller la gamme"=1411, "Vider le flux"=23808, "Vider une file d'attente"=9114, "VISA Assert Interrupt Signal"=2309, "VISA Assert Trigger"=1929, "VISA Assert Utility Signal"=2310, "VISA Clear"=1927, "VISA Close"=1922, "VISA Disable Event"=1940, "VISA Discard Events"=1941, "VISA Enable Event"=1942, "VISA Find Resource"=1923, "VISA Flush I/O Buffer"=2302, "VISA GPIB Command"=2315, "VISA GPIB Control ATN"=2316, "VISA GPIB Control REN"=2304, "VISA GPIB Pass Control"=2317, "VISA GPIB Send IFC"=2318, "VISA In 16"=1930, "VISA In 32"=1944, "VISA In 64"=2140, "VISA In 8"=1936, "VISA Lock"=1993, "VISA Map Address"=1932, "VISA Map Trigger"=2311, "VISA Memory Allocation"=1997, "VISA Memory Allocation Ex"=2146, "VISA Memory Free"=1998, "VISA Move"=2303, "VISA Move In 16"=1948, "VISA Move In 32"=1991, "VISA Move In 64"=2144, "VISA Move In 8"=1946, "VISA Move Out 16"=1949, "VISA Move Out 32"=1992, "VISA Move Out 64"=2145, "VISA Move Out 8"=1947, "VISA Open"=2308, "VISA Out 16"=1931, "VISA Out 32"=1945, "VISA Out 64"=2141, "VISA Out 8"=1937, "VISA Peek 16"=1934, "VISA Peek 32"=1995, "VISA Peek 64"=2142, "VISA Peek 8"=1938, "VISA Poke 16"=1935, "VISA Poke 32"=1996, "VISA Poke 64"=2143, "VISA Poke 8"=1939, "VISA Read"=1925, "VISA Read STB"=1928, "VISA Read To File"=2313, "VISA Refnum en session"=2300, "VISA Set I/O Buffer Size"=2301, "VISA Status Description"=1924, "VISA Unlock"=1994, "VISA Unmap Address"=1933, "VISA Unmap Trigger"=2312, "VISA USB Control In"=2086, "VISA USB Control Out"=2087, "VISA VXI Cmd or Query"=2305, "VISA Wait On Event"=1943, "VISA Write"=1926, "VISA Write From File"=2314, "Vitesse de la lumière dans le vide (m/s)"=23518, "Vérificateur de soupape"=3833, "Wait for GPIB RQS"=1952, "WaitSRQ"=1990, "Échangeur"=3828, "Écrire dans un fichier"=1408, "Écrire dans un fichier journal LabVIEW"=8079, "Écrire plusieurs éléments dans le flux"=23804, "Écrire sur un périphérique"=1431, "Écrire sur une FIFO RT"=24002, "Écrire un seul élément dans le flux"=23798, "Écrire une variable"=23782, "Écrire une variable avec timeout"=23789, "Écriture directe de la variable "=23788, "Écriture par balayage de la variable"=23787, "Égal à 0 ?"=1113, "Égalité des nombres à virgule flottante ?"=23064, "Égaux ?"=1102, "Élément de menu sélectionné"=9001, "Élément utilisateur"=3506, "Établir une connexion à une variable"=23779, "Établir une connexion à une variable en arrière-plan"=23791, "État"=2198, "État de la fenêtre d'aide"=1354, "Étiquette libre"=2321]
          w107 = refnum<vi> refnum  # While循环
          w109 = 2003 items=[" Additionner (avec terminaux d'erreur)"=3915, " Arbre (classique)"=21819, " Arbre (moderne)"=21793, " Arbre (système)"=21794, " Barre de défil. horiz. de dlg"=21905, " Barre de défil. vert. de dlg"=21906, " Barre de progression horizontale (moderne)"=21102, " Barre de progression horizontale (système)"=21910, " Barre de progression verticale (moderne)"=21104, " Barre de progression verticale (système)"=21909, " Bin 1"=3073, " Bin 2"=21755, " Boucle While 1"=2003, " Boucle While 2"=2352, " Bouton Annuler (moderne)"=21739, " Bouton Annuler (système)"=3131, " Bouton OK (moderne)"=21738, " Bouton OK (système)"=3130, " Bouton radio (système)"=3133, " Bouton rotatif (classique)"=3005, " Bouton rotatif (moderne)"=21000, " Bouton-poussoir carré"=3119, " Bouton-poussoir carré (profil)"=3113, " Bouton-poussoir circulaire"=3118, " Bouton-poussoir circulaire (profil)"=3112, " Boutons radio (classique)"=22003, " Boutons radio (moderne)"=22001, " Boutons radio (système)"=22002, " Boîte de couleur encadrée (classique)"=3008, " Boîte de couleur encadrée (moderne)"=21019, " Boîte de dialogue de fichier (obsolète)"=8081, " Boîte en relief (classique)"=3600, " Boîte en relief (moderne)"=3637, " Boîte épaisse (encastrée)"=3635, " Cadran (classique)"=3050, " Cadran (moderne)"=21732, " Cadre encastré (moderne)"=3607, " Cadre encastré (système)"=3624, " Case à cocher (classique)"=3117, " Case à cocher (moderne)"=21924, " Case à cocher (système)"=3132, " Case à cocher mixte (système)"=21333, " Chaîne de dlg"=2110, " Chaîne déroulante (classique)"=3304, " Chaîne déroulante (moderne)"=21604, " Chaîne déroulante (système)"=21917, " Cluster (classique)"=3400, " Cluster (moderne)"=21607, " Commande chaîne (classique)"=3200, " Commande chaîne (moderne)"=21701, " Commande chaîne (système)"=21920, " Commande chemin (classique)"=3203, " Commande chemin (moderne)"=21730, " Commande chemin (système)"=21922, " Commande horodatage (classique)"=5555, " Commande horodatage (moderne)"=21913, " Commande horodatage (système)"=21967, " Commande numérique (classique)"=3000, " Commande numérique (moderne)"=21003, " Commande numérique (système)"=21919, " Commande numérique à incrémentation (système)"=21900, " Commande onglets (classique)"=3330, " Commande onglets (moderne)"=3332, " Commande onglets (système)"=3331, " Commande variable partagée (classique)"=3472, " Commande variable partagée (moderne)"=21814, " Copier (obsolète)"=1416, " Coude gauche vers le bas (ombré)"=3711, " Coude gauche vers le bas (plat)"=3811, " Coude gauche vers le haut (ombré)"=3708, " Coude gauche vers le haut (plat)"=3808, " Coude vers le bas à droite (ombré)"=3717, " Coude vers le bas à droite (plat)"=3817, " Coude vers le haut à droite (ombré)"=3714, " Coude vers le haut à droite (plat)"=3814, " Diviser (avec terminaux d'erreur)"=3918, " Données numériques (classique)"=3210, " Données numériques (moderne)"=21216, " Déplacer (obsolète)"=1415, " Entonnoir 1"=21754, " Entonnoir 2"=3072, " Fermer un fichier (obsolète)"=1405, " Glissière horizontale (classique)"=3010, " Glissière horizontale (système)"=21904, " Glissière verticale (système)"=21903, " Glissière à curseur horizontale (classique)"=3011, " Glissière à curseur horizontale (moderne)"=21101, " Glissière à curseur horizontale (système)"=21902, " Glissière à curseur verticale (classique)"=3007, " Glissière à curseur verticale (moderne)"=21017, " Glissière à curseur verticale (système)"=21901, " Glissière à niveau horizontale (classique)"=3012, " Glissière à niveau horizontale (moderne)"=21100, " Glissière à niveau verticale (classique)"=3009, " Glissière à niveau verticale (moderne)"=21014, " Graphe (classique)"=3504, " Graphe (moderne)"=21703, " Graphe d'intensité (classique)"=3510, " Graphe d'intensité (moderne)"=21720, " Graphe déroulant (moderne)"=21717, " Graphe déroulant d'intensité (classique)"=3509, " Graphe déroulant d'intensité (moderne)"=21719, " Graphe numérique (classique)"=3511, " Graphe numérique (moderne)"=21718, " Graphe XY (classique)"=3500, " Graphe XY (moderne)"=21716, " Horodatage (constante du diagramme)"=2068, " Indicateur chaîne (classique)"=3201, " Indicateur chaîne (moderne)"=21702, " Indicateur chemin (classique)"=3204, " Indicateur chemin (moderne)"=21731, " Indicateur horodatage (classique)"=5556, " Indicateur horodatage (moderne)"=21914, " Indicateur numérique (classique)"=3001, " Indicateur numérique (moderne)"=21004, " Infos sur le fichier/répertoire (obsolète)"=1413, " Interface CAN (classique)"=3339, " Interface CAN (constante du diagramme)"=2123, " Interface CAN (moderne)"=21815, " Interface CAN (système)"=21964, " Interrupteur à bascule horizontal (classique)"=3110, " Interrupteur à bascule horizontal (moderne)"=21700, " Interrupteur à bascule vertical (classique)"=3111, " Interrupteur à bascule vertical (moderne)"=21005, " Interrupteur à glissière vertical (classique)"=3115, " Interrupteur à glissière vertical (moderne)"=21741, " Jauge (classique)"=3040, " Jauge (moderne)"=21009, " LED carrée (classique)"=3121, " LED carrée (moderne)"=21013, " LED circulaire (classique)"=3120, " LED circulaire (moderne)"=21012, " Ligne (ciselée, fine)"=3627, " Ligne (ciselée, système)"=3632, " Ligne (ciselée, épaisse)"=3630, " Ligne (fine)"=3626, " Ligne (épaisse)"=3629, " Ligne avec flèche (fine)"=3628, " Ligne avec flèche (épaisse)"=3631, " Liste déroulante (classique)"=21806, " Liste déroulante (moderne)"=21792, " Liste déroulante (système)"=21805, " Liste multicolonne (classique)"=21799, " Liste multicolonne (moderne)"=21791, " Liste multicolonne (système)"=21798, " Menu déroulant (classique)"=3018, " Menu déroulant (moderne)"=21600, " Menu déroulant d'images (classique)"=3015, " Menu déroulant d'images (moderne)"=21602, " Menu déroulant d'images (système)"=21925, " Menu déroulant texte (classique)"=3014, " Menu déroulant texte (constante du diagramme)"=2008, " Menu déroulant texte (moderne)"=21601, " Menu déroulant texte (système)"=3060, " Menu déroulant texte et images (classique)"=3016, " Menu déroulant texte et images (moderne)"=21603, " Mettre à jour le fichier (obsolète)"=1406, " Moteur (ombré)"=3720, " Moteur (plat)"=3820, " Multiplier (avec terminaux d'erreur)"=3917, " Nom d'échelle DAQmx (classique)"=3317, " Nom d'échelle DAQmx (constante du diagramme)"=2116, " Nom d'échelle DAQmx (moderne)"=21775, " Nom d'échelle DAQmx (système)"=21952, " Nom de périphérique DAQmx (classique)"=3318, " Nom de périphérique DAQmx (constante du diagramme)"=2093, " Nom de périphérique DAQmx (moderne)"=21773, " Nom de périphérique DAQmx (système)"=21950, " Nom de ressource VISA (classique)"=3409, " Nom de ressource VISA (moderne)"=21737, " Nom de tâche DAQmx (classique)"=3442, " Nom de tâche DAQmx (constante du diagramme)"=3434, " Nom de tâche DAQmx (moderne)"=21778, " Nom de tâche DAQmx (système)"=21959, " Nom logique IVI (classique)"=3414, " Nom logique IVI (constante du diagramme)"=3420, " Nom logique IVI (moderne)"=21736, " Numérique de dlg 1"=2100, " Numérique de dlg 2"=3006, " Pixmap (attention : dangereux)"=3507, " Point d'E/S FieldPoint (classique)"=3439, " Point d'E/S FieldPoint (constante du diagramme)"=3440, " Point d'E/S FieldPoint (moderne)"=21784, " Pompe vers la droite (ombrée)"=3719, " Pompe vers la droite (plate)"=3819, " Pompe vers la gauche (ombrée)"=3713, " Pompe vers la gauche (plate)"=3813, " RecomposerRéfValDonnéesDéverrou (warning: dangerous)"=2407, " RecomposerVariant (warning: dangerous)"=2405, " Rectangle de couleur (brisé ?)"=3625, " Ressource Motion (classique)"=3448, " Ressource Motion (constante du diagramme)"=3449, " Ressource Motion (moderne)"=21787, " Réservoir (classique)"=3020, " Réservoir (moderne)"=21006, " Réservoir atmosphérique (classique)"=3070, " Réservoir atmosphérique (moderne)"=21751, " Réservoir de pression (ombré)"=21753, " Réservoir de pression (plat)"=3075, " Réservoir ouvert (ombré classique)"=3074, " Réservoir ouvert (plat classique)"=21752, " Soupape courbée vers la droite (contour)"=3805, " Soupape courbée vers la droite (ombrée)"=21765, " Soupape courbée vers la droite (plate)"=3705, " Soupape courbée vers la gauche (contour)"=3801, " Soupape courbée vers la gauche (ombrée)"=21761, " Soupape courbée vers la gauche (plate)"=3701, " Soupape courbée vers le bas (contour)"=3807, " Soupape courbée vers le bas (ombrée)"=21767, " Soupape courbée vers le bas (plate)"=3707, " Soupape courbée vers le haut (contour)"=3803, " Soupape courbée vers le haut (ombrée)"=21763, " Soupape courbée vers le haut (plate)"=3703, " Soupape rectangulaire vers la droite (contour)"=3804, " Soupape rectangulaire vers la droite (ombrée)"=21764, " Soupape rectangulaire vers la droite (plate)"=3704, " Soupape rectangulaire vers la gauche (contour)"=3800, " Soupape rectangulaire vers la gauche (ombrée)"=21760, " Soupape rectangulaire vers la gauche (plate)"=3700, " Soupape rectangulaire vers le bas (contour)"=3806, " Soupape rectangulaire vers le bas (ombrée)"=21766, " Soupape rectangulaire vers le bas (plate)"=3706, " Soupape rectangulaire vers le haut (contour)"=21762, " Soupape rectangulaire vers le haut (ombrée)"=3802, " Soupape rectangulaire vers le haut (plate)"=3702, " Source de déclenchement analogique DAQmx (classique)"=3336, " Source de déclenchement analogique DAQmx (constante du diagramme)"=2119, " Source de déclenchement analogique DAQmx (moderne)"=21774, " Source de déclenchement analogique DAQmx (système)"=21951, " Soustraire (avec terminaux d'erreur)"=3916, " Supprimer (obsolète)"=1417, " Switch DAQmx (classique)"=3337, " Switch DAQmx (constante du diagramme)"=2121, " Switch DAQmx (moderne)"=21776, " Switch DAQmx (système)"=21953, " Table (classique)"=21796, " Table (moderne)"=21790, " Table (système)"=21797, " Tableau (classique)"=3300, " Tableau (constante du diagramme)"=2070, " Tableau (moderne)"=21608, " Tag de refnum défini par l'utilisateur (classique)"=3429, " Tag de refnum défini par l'utilisateur (constante du diagramme)"=3426, " Tag de refnum défini par l'utilisateur (moderne)"=21745, " Tag de refnum défini par l'utilisateur aplati (classique)"=3454, " Tag de refnum défini par l'utilisateur aplati (modern)"=21747, " Tag défini par l'utilisateur aplati (moderne)"=21749, " Tag défini par utilisateur (classique)"=3329, " Tag défini par utilisateur (constante du diagramme)"=2114, " Tee vers la droite (ombré)"=3715, " Tee vers la droite (plat)"=3815, " Tee vers la gauche (ombré)"=3709, " Tee vers la gauche (plat)"=3809, " Tee vers le bas (ombré)"=3718, " Tee vers le bas (plat)"=3818, " Tee vers le haut (ombré)"=3712, " Tee vers le haut (plat)"=3812, " Terminal DAQmx (classique)"=3319, " Terminal DAQmx (constante du diagramme)"=2117, " Terminal DAQmx (moderne)"=21781, " Terminal DAQmx (système)"=21955, " Thermomètre (classique)"=3021, " Thermomètre (moderne)"=21007, " Tuyau horiz. (ombré)"=3710, " Tuyau horiz. (plat)"=3810, " Tuyau vertical (ombré)"=3716, " Tuyau vertical (plat)"=3816, " Tâche CAN (classique)"=3470, " Tâche CAN (constante du diagramme)"=3471, " Tâche CAN (moderne)"=21789, " Tâche CAN (système)"=21963, " Voie CAN (classique)"=3340, " Voie CAN (constante du diagramme)"=2124, " Voie CAN (moderne)"=21817, " Voie CAN (système)"=21966, " Voie de NI-DAQ traditionnel (classique)"=3320, " Voie de NI-DAQ traditionnel (constante du diagramme)"=2085, " Voie de NI-DAQ traditionnel (moderne)"=21733, " Voie globale DAQmx (classique)"=3443, " Voie globale DAQmx (constante du diagramme)"=3430, " Voie globale DAQmx (moderne)"=21770, " Voie globale DAQmx (système)"=21957, " Voie physique DAQmx (classique)"=3335, " Voie physique DAQmx (constante du diagramme)"=2118, " Voie physique DAQmx (moderne)"=21777, " Voie physique DAQmx (système)"=21954, " Vumètre (classique)"=3030, " Vumètre (moderne)"=21008, " Écrire dans un fichier binaire"=8078, " Écrire dans un fichier texte"=8080, " Énum (classique)"=3023, " Énum (moderne)"=21605, " Énum (système)"=3062, " Étiquette (moderne)"=21960, " Étiquette (système)"=21961, "Activer le repérage des menus"=9002, "Adapter d'entier à virgule fixe"=5567, "Adapter de virgule fixe à entier"=5566, "Adapter le type"=1166, "Additionner"=1050, "Additionner les éléments du tableau"=1903, "Agitateur"=3831, "Ajouter la chaîne Vrai/Faux"=1511, "Ajouter un élément au début d'une file d'attente"=9129, "Ajouter un élément à la fin d'une file d'attente"=9111, "Ajouter un élément à la fin d'une file d'attente avec pertes"=9130, "Ajouter une chaîne multiligne"=1510, "AllSpoll"=1960, "Ampoule carrée"=3105, "Ampoule circulaire"=3104, "Ancien VISA Open"=1921, "Annuler une notification"=9107, "Aperçu du premier élément d'une file d'attente"=9112, "Aplatir en chaîne"=1164, "Aplatir en XML"=8400, "Appel par référence MathScript"=3906, "Appeler la méthode parente"=2354, "Appeler par référence"=3901, "Appeler une fonction d'une DLL"=2062, "Arc cosinus"=1207, "Arc cosinus hyperbolique"=1218, "Arc cosécante"=23050, "Arc cosécante hyperbolique"=23056, "Arc cotangente"=23052, "Arc cotangente hyperbolique"=23058, "Arc sinus"=1206, "Arc sinus hyperbolique"=1217, "Arc sécante"=23051, "Arc sécante hyperbolique"=23057, "Arc tangente"=1208, "Arc tangente (2 entrées)"=1228, "Arc tangente hyperbolique"=1219, "Array Interface Control"=23777, "Arrondir vers +l'infini"=1076, "Arrondir vers -l'infini"=1075, "Arrondir à l'entier le plus proche"=1055, "Arrêter"=1350, "Assembler"=2049, "Assembler des signaux"=2350, "Assembler par nom"=2057, "Attendre (ms)"=1302, "Attendre un multiple de ms"=1327, "Attendre une activité sur la face-avant"=1328, "Attendre une notification"=9105, "Attendre une notification avec historique des notificateurs"=9131, "Attendre une notification de plusieurs"=9106, "Attendre une notification de plusieurs avec historique des notificateurs"=9132, "Attendre une occurrence"=1701, "Attente d'activité"=1722, "Automation Fermer"=8001, "Automation Ouvrir"=8000, "Balayer un fichier"=2082, "Balayer une chaîne"=2080, "Balayer une valeur"=1534, "Barre de division horizontale"=21861, "Barre de division horizontale (classique)"=21863, "Barre de division horizontale (système)"=21865, "Barre de division verticale"=21860, "Barre de division verticale (classique)"=21862, "Barre de division verticale (système)"=21864, "Barre de défilement horizontale"=21110, "Barre de défilement verticale"=21111, "Barre de menus du VI actuel"=9000, "Barre graduée horizontale"=21106, "Barre graduée verticale"=21107, "Base du logarithme népérien"=23510, "Bibliothèque de VIs"=1425, "Bitpack en tableau"=3135, "Bluetooth - Attendre un récepteur"=9147, "Bluetooth - Créer un récepteur"=9151, "Bluetooth - Découvrir"=9152, "Bluetooth - Fermer la connexion"=9148, "Bluetooth - Lire"=9149, "Bluetooth - Ouvrir une connexion"=9153, "Bluetooth - Écrire"=9150, "Booléen en (0,1)"=1167, "Boucle cadencée"=5570, "Boucle de contrôle et simulation"=2099, "Boucle For"=2002, "Bouton allongé à étiquette"=3125, "Bouton carré"=3101, "Bouton carré plat"=3103, "Bouton carré plat de plate-forme"=3134, "Bouton carré à étiquette"=3123, "Bouton circulaire"=3100, "Bouton circulaire à étiquette"=3122, "Bouton LED"=3116, "Bouton radio carré"=3107, "Bouton radio circulaire"=3106, "Bouton rectangulaire à étiquette"=3124, "Bouton rond plat"=3102, "Bouton Stop"=21230, "Bouton Stop circulaire"=3127, "Bouton Stop rectangulaire"=3128, "Bouton Texte"=21015, "Bouton-poussoir"=21001, "Boîte arrondie en relief"=3609, "Boîte arrondie encastrée"=3638, "Boîte arrondie encastrée 1"=3610, "Boîte arrondie plate"=3611, "Boîte bouton horizontale"=3636, "Boîte de calcul"=2004, "Boîte de couleur"=3013, "Boîte de couleur à bord mince"=2905, "Boîte de dialogue de fichier"=8058, "Boîte de dialogue à deux boutons"=1341, "Boîte de dialogue à un bouton"=1340, "Boîte encastrée"=3601, "Boîte lisse horizontale"=3633, "Boîte lisse verticale"=3634, "Boîte plate"=3602, "Cadre en relief"=3606, "Cadre plat"=3608, "Carré"=23059, "Casting dynamique d'interface FPGA"=5690, "Cercle en relief"=3603, "Cercle encastré"=3604, "Cercle plat"=3605, "Changer les bases d'unités"=1079, "Charge élémentaire (C)"=23517, "Chaîne aplatie en variant"=8202, "Chaîne au format tableur en tableau"=1539, "Chaîne d'appel"=1999, "Chaîne de date/heure"=1600, "Chaîne décimale en nombre"=1184, "Chaîne en chemin"=1078, "Chaîne en IP"=1711, "Chaîne en tableau d'octets"=1608, "Chaîne en variable partagée"=1830, "Chaîne Fract/Exp en nombre"=1187, "Chaîne hexadécimale en nombre"=1185, "Chaîne octale en nombre"=1186, "Chaîne simple"=2115, "Chemin du VI actuel"=1426, "Chemin en chaîne"=1077, "Chemin en tableau de chaînes"=1423, "Chemin/Chaîne vide ?"=1112, "Chiffre décimal ?"=1119, "Chiffre hexa ?"=1123, "Chiffre octal ?"=1129, "Classe lexicale"=1126, "Classer un tableau 1D"=1120, "Cluster en tableau"=1169, "Code Interface Node"=2050, "Commande Plug-In"=21820, "Commande/état du périphérique"=1433, "Complexe conjugué"=1048, "Complexe en polaire"=1045, "Complexe en Réel/Im"=1044, "Composer un chemin"=1419, "Compresseur"=3832, "Compteur d'impulsions d'horloge (ms)"=1300, "Concaténer des chaînes"=2040, "Constante 'Pas un chemin'"=23524, "Constante 'Pas un refnum'"=23526, "Constante boîte de couleur"=2120, "Constante chaîne"=2007, "Constante chaîne déroulante"=2088, "Constante chaîne vide"=23503, "Constante chemin"=2009, "Constante chemin vide"=23523, "Constante cluster"=2071, "Constante d'Avogadro (1/mol)"=23520, "Constante de Planck (J/Hz)"=23516, "Constante de Rydberg (1/m)"=23521, "Constante de spécification de classe"=2094, "Constante de spécification de classe de variable"=2106, "Constante des gaz parfaits (J/(mol K))"=23522, "Constante Faux"=2006, "Constante fin de ligne"=23525, "Constante gravitationnelle"=23519, "Constante menu déroulant d'erreurs"=2039, "Constante menu déroulant de symboles"=2038, "Constante Nom de variable"=3478, "Constante numérique"=2005, "Constante Retour chariot"=23500, "Constante Retour à la ligne"=23501, "Constante référence de valeur de données"=24134, "Constante tabulation"=23502, "Constante variable partagée"=3473, "Constante énumération"=2090, "Construire un tableau"=2041, "Construire un tableau de clusters"=2047, "Construire une matrice"=8500, "Construire une waveform"=2066, "Conteneur .NET"=2125, "Conteneur ActiveX"=2072, "Contraindre au type"=2402, "Contrôle de l'aide en ligne"=1355, "Contrôle de la fenêtre d'aide"=1353, "Convertir une unité"=2059, "Copier"=8053, "Correspondance de chaîne Vrai/Faux"=1533, "Cosinus"=1201, "Cosinus hyperbolique"=1215, "Cosécante"=1204, "Cosécante hyperbolique"=23053, "Cotangente"=1205, "Cotangente hyperbolique"=23055, "Créer l'extrémité d'écriture d'un flux réseau"=23810, "Créer l'extrémité de lecture d'un flux réseau"=23811, "Créer un dossier"=8055, "Créer un flux"=23796, "Créer un événement utilisateur"=2073, "Créer une FIFO RT"=24000, "Culbuteur"=21002, "Culbuteur vertical"=21740, "Dans la gamme"=1127, "DataSocket Fermer"=1085, "DataSocket Lire"=1086, "DataSocket Ouvrir"=1084, "DataSocket Écrire"=1087, "Date et heure en secondes"=1303, "Date/heure en secondes"=1308, "Demander une désallocation"=1610, "DevClear"=1961, "DevClearList"=1962, "Diagramme d'états"=2051, "Diffuser la référence de valeur Variant"=2410, "Différent de 0 ?"=1116, "Différents ?"=1105, "Dimensionner le handle"=1603, "Distributeur rotatif"=3830, "Diviser"=1053, "Diviser un tableau 1D"=1908, "Droits d'accès"=1412, "Décalage logique"=1081, "Décimer un tableau 1D"=2046, "Décomposer un chemin"=1420, "DécomposerRéfValDonnéesVerrou"=2406, "DécomposerTableau"=2412, "DécomposerVariant"=2404, "Découper un nombre"=1170, "Décrémenter"=1058, "Défaire un package de matrice"=23000, "Définir des éléments de matrice"=8505, "Définir la position dans le fichier"=8073, "Définir la position dans le fichier journal LabVIEW"=8072, "Définir la taille du fichier"=8074, "Définir le nombre d'enregistrements"=8075, "Définir le type et le créateur"=8077, "Définir les autorisations"=8076, "Définir les infos de l'élément de menu"=9006, "Définir un attribut de variant"=8204, "Définir un attribut de waveform"=8207, "Définir une diagonale de matrice"=8504, "Définir une occurrence"=1702, "Définir une sous-matrice"=8506, "Dépassement des données à virgule fixe ?"=5565, "Déplacer"=8068, "Désassembler"=2048, "Désassembler des signaux"=2351, "Désassembler par nom"=2058, "Désenregistrement aux événements"=2076, "Détruire une extrémité d'un flux"=23794, "Effacer l'état de dépassement de virgule fixe"=5562, "En chaîne de sonde"=2413, "En complexe double précision"=1152, "En complexe précision étendue"=1154, "En complexe simple précision"=1151, "En entier de type octet"=1140, "En entier long"=1142, "En entier long non signé"=1145, "En entier mot"=1141, "En entier mot non signé"=1144, "En entier octet non signé"=1143, "En entier quad"=1155, "En entier quad non signé"=1156, "En flottant double précision"=1147, "En flottant précision étendue"=1149, "En flottant simple précision"=1146, "En horodatage"=5560, "En majuscules"=1188, "En minuscules"=1189, "En une classe plus générique"=8017, "En une classe plus spécifique"=8016, "En variant"=8201, "En variant OLE"=8002, "En virgule fixe"=5561, "EnableLocal"=1963, "EnableRemote"=1964, "Enregistrement à des événements"=2065, "Enregistrer un VI Callback d'événement"=2078, "Entrelacer des tableaux 1D"=2045, "Envoyer une notification"=9104, "EOF"=1410, "Epsilon machine"=23528, "Espace blanc ?"=1125, "ET"=1061, "ET logique entre les éléments du tableau"=1911, "Exponentielle"=1211, "Exponentielle (Arg) -1"=1222, "Face-avant secondaire"=21810, "Face-avant secondaire (classique)"=21811, "Face-avant secondaire (système)"=21823, "Faire un package de matrice"=23001, "Fermer un fichier"=8052, "Fermer une connexion à une variable"=23783, "Fermer une référence"=8011, "Fichier TDMS"=3477, "FindLstn"=1965, "FindRQS"=1966, "Flèche droite"=3825, "Flèche gauche"=3826, "Flèche vers le bas"=3824, "Flèche vers le haut"=3823, "Formater dans un fichier"=2083, "Formater en chaîne"=2081, "Formater la chaîne de date/heure"=8100, "Formater une valeur"=1512, "Four"=3829, "Fourche"=2194, "Fusionner les erreurs"=2147, "Glissière horizontale simple"=3003, "Glissière verticale"=3004, "Glissière verticale simple"=3002, "GPIB Clear"=1954, "GPIB Initialization"=1957, "GPIB Misc"=1956, "GPIB Read"=1951, "GPIB Serial Poll"=1955, "GPIB Status"=1959, "GPIB Trigger"=1953, "GPIB Wait"=1958, "GPIB Write"=1950, "Graphe de signaux mixte"=21721, "Graphe déroulant"=3501, "Graphe déroulant 1"=21010, "Générer un événement de suivi défini par l'utilisateur"=2250, "Générer un événement utilisateur"=2074, "Générer une activité sur la face-avant"=1329, "Générer une occurrence"=1700, "Handle Peek"=1604, "Handle Poke"=1605, "ID du processeur actuel"=24131, "Image 2D"=3508, "Image 3D"=23776, "Implique"=1080, "Imprimable ?"=1124, "Inclure l'état de dépassement de virgule fixe"=5564, "Incrémenter"=1057, "Indexer et assembler un tableau de clusters"=2056, "Indexer un tableau"=2042, "Indexer un tableau de chaînes"=1531, "Indice de ressource"=1088, "Informations sur le processeur"=24130, "Infos sur le fichier/répertoire"=8082, "Infos sur le volume"=1414, "Infos sur un raccourci de menu"=9007, "Infos sur un élément de menu"=9005, "Inférieur ?"=1111, "Inférieur ou égal ?"=1104, "Inférieur ou égal à 0 ?"=1115, "Inférieur à 0 ?"=1118, "Initialiser un tableau"=2053, "Inlining du nœud C"=2104, "Insérer dans un tableau"=3911, "Insérer des éléments de menu"=9003, "Interdire l'accès"=8057, "Interpoler un tableau 1D"=1905, "Interrupteur horizontal"=3108, "Interrupteur vertical"=3109, "Interrupteur à glissière"=21011, "Interrupteur à glissière horizontal"=3114, "Inverse de e"=23511, "Inverse de Pi"=23507, "Inverser"=1059, "Inverser un tableau 1D"=1900, "Inverser une chaîne"=1537, "IP en chaîne"=1710, "IrDA Attendre un récepteur"=9143, "IrDA Créer un récepteur"=9140, "IrDA Découvrir"=9141, "IrDA Fermer la connexion"=9144, "IrDA Lire"=9145, "IrDA Ouvrir une connexion"=9142, "IrDA Écrire"=9146, "Jauge pour Simon"=32600, "Joint"=2195, "Jonction"=2197, "Lecture directe de la variable "=23785, "Lecture par balayage de la variable"=23784, "Libérer un notificateur"=9102, "Libérer une file d'attente"=9109, "Ligne horiz."=3821, "Ligne verticale"=3822, "Lire plusieurs éléments du flux"=23803, "Lire un fichier"=1407, "Lire un fichier binaire"=8051, "Lire un fichier binaire avec préallocation"=24135, "Lire un fichier journal LabVIEW"=8069, "Lire un fichier texte"=8070, "Lire un périphérique"=1432, "Lire un seul élément du flux"=23797, "Lire une FIFO RT"=24001, "Lire une variable"=23781, "Lire une variable avec timeout"=23786, "Lister le contenu d'un répertoire"=1418, "Lister le contenu du dossier"=8083, "Logarithme base 10 de e"=23512, "Logarithme en base 10"=1210, "Logarithme en base 2"=1225, "Logarithme en base X"=1224, "Logarithme népérien"=1209, "Logarithme népérien (Arg +1)"=1221, "Logarithme népérien de 10"=23513, "Logarithme népérien de 2"=23514, "Logarithme népérien de Pi"=23508, "Longueur d'une chaîne"=1502, "MakeAddr"=1967, "Mantisse et exposant"=1150, "Max. et min."=1108, "Max. et min. d'un tableau"=1907, "Menu déroulant"=3061, "Menu déroulant d'attribut du tag"=2063, "Menu déroulant en retrait"=3019, "Menu déroulant popup"=3017, "Mettre à jour le fichier"=8059, "Moins l'infini"=23509, "Multiplier"=1052, "Multiplier les éléments du tableau"=1904, "Multiplier par une puissance de 2"=1074, "Ne pas diffuser la référence de valeur Variant"=2411, "Nom de ressource VISA"=3421, "Nombre aléatoire (0-1)"=1070, "Nombre de niveaux du cache"=24133, "Nombre en chaîne au format ingénieur"=1183, "Nombre en chaîne décimale"=1180, "Nombre en chaîne exponentielle"=1505, "Nombre en chaîne fractionnaire"=1506, "Nombre en chaîne hexadécimale"=1181, "Nombre en chaîne octale"=1182, "Nombre en tableau de booléens"=1814, "Non"=1064, "Non ET"=1071, "Non OU"=1072, "Non OU exclusif"=1073, "Nouveau fichier"=1404, "Nouveau répertoire"=1402, "Nouveau VI"=8014, "Nouvel objet de VI"=8015, "Nouvelle référence de valeur de données"=2408, "Nouvelle session IVI"=8102, "Numérique simple"=2900, "Nœud d'expression"=2201, "Nœud de données d'événement"=2102, "Nœud de méthode"=3900, "Nœud de propriété"=1920, "Nœud de rétroaction"=2353, "Nœud du constructeur"=3904, "Nœud MathScript"=2357, "Objet LabVIEW"=3457, "Obtenir des composantes à virgule fixe"=11163, "Obtenir l'état d'un notificateur"=9103, "Obtenir l'état d'une file d'attente"=9110, "Obtenir la diagonale d'une matrice"=8501, "Obtenir la position dans le fichier"=8062, "Obtenir la position dans le fichier journal LabVIEW"=8061, "Obtenir la taille du fichier"=8063, "Obtenir le nombre d'enregistrements"=8064, "Obtenir le type et le créateur"=8066, "Obtenir les autorisations"=8065, "Obtenir les composantes d'une waveform"=2067, "Obtenir les données glissées et déposées"=9154, "Obtenir les infos sur le volume"=8067, "Obtenir les éléments d'une matrice"=8502, "Obtenir un attribut de variant"=8205, "Obtenir un attribut de waveform"=8208, "Obtenir un notificateur"=9101, "Obtenir une file d'attente"=9108, "Obtenir une sous-matrice"=8503, "Opposé"=1069, "Opérateur arithmétique"=2200, "OU"=1062, "OU exclusif"=1063, "OU logique entre les éléments du tableau"=1910, "Ouvrir et vérifier la connexion d'une variable"=23790, "Ouvrir un fichier"=1403, "Ouvrir un périphérique"=1430, "Ouvrir une référence d'application"=8012, "Ouvrir une référence d'objet de VI"=8013, "Ouvrir une référence de VI"=8010, "Ouvrir/Créer/Remplacer un fichier"=8050, "Ouvrir/Créer/Remplacer un fichier journal LabVIEW"=8054, "Ovale lissé"=32500, "Ovale ombré"=32509, "Ovale à gradient horizontal"=32502, "Ovale à gradient vertical"=32501, "Partie de bouton"=21020, "Pas un nombre/chemin/refnum ?"=1128, "Pas une variable partagée"=23527, "PassControl"=1968, "Permuter les mots"=1163, "Permuter les octets"=1162, "Permuter les valeurs"=2401, "Permuter les éléments de vecteur"=1912, "Pi"=23504, "Pi / 2"=23506, "Pi x 2"=23505, "Pixmap"=3505, "Plus l'infini"=23515, "Polaire en complexe"=1047, "Polaire en Réel/Im"=23061, "PPoll"=1969, "PPollConfig"=1970, "PPollUnconfig"=1971, "Premier appel ?"=1083, "Préserver la classe à l'exécution"=8018, "Puissance de 10"=1212, "Puissance de 2"=1223, "Puissance de X"=1213, "Quitter LabVIEW"=1352, "Quotient et Reste"=1056, "Racine carrée"=1060, "Racine y-ième de x"=23062, "Rampe de couleur"=3022, "RcvRespMsg"=1972, "ReadStatus"=1973, "Receive"=1974, "ReceiveSetup"=1975, "Rechercher"=1409, "Rechercher dans un conteneur de variables"=23802, "Rechercher dans un tableau 1D"=1901, "Rechercher des symboles"=8101, "Rechercher et remplacer une chaîne"=3914, "Rechercher la première occurrence"=1532, "Rechercher une expression"=1535, "Rechercher/Découper une chaîne"=1538, "RecomperTableau"=2403, "Rectangle arrondi lissé"=32505, "Rectangle arrondi ombré"=32508, "Rectangle arrondi à gradient horizontal"=32507, "Rectangle arrondi à gradient vertical"=32506, "Rectangle à gradient horizontal"=32504, "Rectangle à gradient vertical"=32503, "Redimensionner un tableau"=2055, "Redimensionner une matrice"=8508, "Redresser à partir d'une chaîne"=1165, "Redresser à partir d'XML"=8401, "Refnum Automation"=3410, "Refnum d'application"=3412, "Refnum d'occurrence"=3406, "Refnum DataSocket"=3417, "Refnum de .NET"=3441, "Refnum de Callback d'événement"=3435, "Refnum de commande"=3419, "Refnum de connexion réseau Bluetooth"=3468, "Refnum de connexion réseau IrDA"=3450, "Refnum de connexion réseau TCP"=3407, "Refnum de connexion réseau UDP"=3418, "Refnum de fichier journal LabVIEW"=3402, "Refnum de fichier à flux d'octets"=3408, "Refnum de FIFO"=3474, "Refnum de file d'attente"=3424, "Refnum de menu"=3413, "RefNum de notificateur"=3423, "Refnum de périphérique"=3405, "Refnum de VI"=3422, "Refnum défini par l'utilisateur"=3428, "Refnum en chemin"=1424, "Refnum en session"=2306, "Refnum FPGA en session"=2322, "Regrouper des nombres"=1171, "Remplacer une portion d'un tableau"=3910, "Remplacer une portion de chaîne"=3913, "ResetSys"=1976, "Rotation"=1082, "Rotation dans un tableau 1D"=1906, "Rotation dans une chaîne"=1536, "Rotation droite avec retenue"=1607, "Rotation gauche avec retenue"=1606, "Réel/Im en complexe"=1046, "Réel/Im en polaire"=23060, "Référence de valeur de données"=3476, "Référence de VI Serveur"=2091, "Référence de VI statique"=2084, "Région"=2196, "Répertoire par défaut"=1427, "Répertoire temporaire"=1435, "Réservoir horizontal"=3071, "Script MATLAB"=9020, "Secondes en date/heure"=1309, "Send"=1977, "SendCmds"=1978, "SendDataBytes"=1979, "SendIFC"=1980, "SendList"=1981, "SendLLO"=1982, "SendSetup"=1983, "Session d'enregistrement"=2319, "Session en refnum"=2307, "Session IMAQ"=3415, "Session non enregistrée"=2320, "SetRWLS"=1984, "SetTimeOut"=1985, "Seuil d'un tableau 1D"=1909, "Signe"=1049, "Sinc"=1227, "Sinus"=1200, "Sinus et cosinus"=1220, "Sinus hyperbolique"=1214, "Sous-ensemble d'un tableau"=2044, "Sous-ensemble d'une chaîne"=1503, "Soustraire"=1051, "Structure Condition"=2001, "Structure multifréquence"=2199, "Structure Séquence déroulée"=2069, "Structure Séquence empilée"=2000, "Structure à conditions désactivées"=2064, "Structure à diagrammes désactivés"=2054, "Structure Élément en place"=2360, "Structure Événement"=2052, "Supprimer"=8056, "Supprimer des éléments de menu"=9004, "Supprimer l'état de dépassement de virgule fixe"=5563, "Supprimer la session IVI"=8103, "Supprimer le premier élément d'une file d'attente"=9113, "Supprimer un attribut de variant"=8206, "Supprimer un attribut de waveform"=8209, "Supprimer un événement utilisateur"=2075, "Supprimer une FIFO RT"=24003, "Supprimer une portion d'un tableau"=3912, "Supprimer une référence de valeur de données"=2409, "Supérieur ?"=1110, "Supérieur ou égal ?"=1103, "Supérieur ou égal à 0 ?"=1114, "Supérieur à 0 ?"=1117, "Sécante"=1203, "Sécante hyperbolique"=23054, "Sélectionner"=1516, "Séquence cadencée"=5573, "Tableau bitpack en données"=3136, "Tableau d'octets en chaîne"=1609, "Tableau de booléens en nombre"=1815, "Tableau de chaînes en chemin"=1422, "Tableau en chaîne au format tableur"=1540, "Tableau en cluster"=1168, "Tableau vide ?"=23063, "Taille d'un tableau"=1809, "Taille de matrice"=8507, "Taille du cache de données"=24132, "Tangente"=1202, "Tangente hyperbolique"=1216, "Tapis roulant"=3827, "TCP Attendre un récepteur"=1712, "TCP Créer un récepteur"=1717, "TCP Fermer la connexion"=1713, "TCP Lire"=1716, "TCP Lire des données Flex"=1720, "TCP Lire des données plates"=1718, "TCP Ouvrir une connexion"=1715, "TCP Écrire"=1714, "TCP Écrire des données Flex"=1721, "TCP Écrire des données plates"=1719, "TDMS - Configurer des lectures asynchrones (réf de données)"=2153, "TDMS - Configurer des écritures asynchrones (réf de données)"=2152, "TDMS - Lecture asynchrone (Avancée) (réf de données)"=2151, "TDMS - Obtenir l'état des lectures asynchrones (réf de données)"=2155, "TDMS - Obtenir l'état des écritures asynchrones (réf de données)"=2154, "TDMS - Écriture asynchrone (Avancée) (réf de données)"=2150, "TDMS Close"=24113, "TDMS Defragment"=24119, "TDMS Flush"=24117, "TDMS Get Properties"=24115, "TDMS List Contents"=24116, "TDMS Open"=24112, "TDMS Read"=24111, "TDMS Refnum To File ID"=24120, "TDMS Set Properties"=24114, "TDMS Write"=24110, "TDMS Write IP"=24118, "TestSRQ"=1986, "TestSys"=1987, "Texte en UTF-8"=23066, "Toujours copier"=2400, "Transposer un tableau 1D"=23068, "Transposer un tableau 2D"=1902, "Transposée d'une matrice"=8509, "Triangle en relief vers la droite"=3613, "Triangle en relief vers la gauche"=3612, "Triangle en relief vers le bas"=3615, "Triangle en relief vers le haut"=3614, "Triangle encastré vers la droite"=3617, "Triangle encastré vers la gauche"=3616, "Triangle encastré vers le bas"=3619, "Triangle encastré vers le haut"=3618, "Triangle plat vers la droite"=3621, "Triangle plat vers la gauche"=3620, "Triangle plat vers le bas"=3623, "Triangle plat vers le haut"=3622, "Trier un tableau de chaînes"=23065, "Trigger"=1988, "TriggerList"=1989, "Tuyau à plusieurs segments"=23780, "Type de chemin"=1421, "Type et créateur"=1434, "UDP Fermer"=1726, "UDP Lire"=1724, "UDP Multicast - Ouvrir"=1727, "UDP Ouvrir"=1723, "UDP Écrire"=1725, "UTF-8 en texte"=23067, "Valeur absolue"=1054, "Variable globale"=2060, "Variable locale"=2061, "Variable partagée"=23778, "Variable partagée en chaîne"=1831, "Variant"=3310, "Variant en chaîne aplatie"=8203, "Variant en donnée"=8003, "Variant OLE"=3150, "Verrouiller la gamme"=1411, "Vider le flux"=23808, "Vider une file d'attente"=9114, "VISA Assert Interrupt Signal"=2309, "VISA Assert Trigger"=1929, "VISA Assert Utility Signal"=2310, "VISA Clear"=1927, "VISA Close"=1922, "VISA Disable Event"=1940, "VISA Discard Events"=1941, "VISA Enable Event"=1942, "VISA Find Resource"=1923, "VISA Flush I/O Buffer"=2302, "VISA GPIB Command"=2315, "VISA GPIB Control ATN"=2316, "VISA GPIB Control REN"=2304, "VISA GPIB Pass Control"=2317, "VISA GPIB Send IFC"=2318, "VISA In 16"=1930, "VISA In 32"=1944, "VISA In 64"=2140, "VISA In 8"=1936, "VISA Lock"=1993, "VISA Map Address"=1932, "VISA Map Trigger"=2311, "VISA Memory Allocation"=1997, "VISA Memory Allocation Ex"=2146, "VISA Memory Free"=1998, "VISA Move"=2303, "VISA Move In 16"=1948, "VISA Move In 32"=1991, "VISA Move In 64"=2144, "VISA Move In 8"=1946, "VISA Move Out 16"=1949, "VISA Move Out 32"=1992, "VISA Move Out 64"=2145, "VISA Move Out 8"=1947, "VISA Open"=2308, "VISA Out 16"=1931, "VISA Out 32"=1945, "VISA Out 64"=2141, "VISA Out 8"=1937, "VISA Peek 16"=1934, "VISA Peek 32"=1995, "VISA Peek 64"=2142, "VISA Peek 8"=1938, "VISA Poke 16"=1935, "VISA Poke 32"=1996, "VISA Poke 64"=2143, "VISA Poke 8"=1939, "VISA Read"=1925, "VISA Read STB"=1928, "VISA Read To File"=2313, "VISA Refnum en session"=2300, "VISA Set I/O Buffer Size"=2301, "VISA Status Description"=1924, "VISA Unlock"=1994, "VISA Unmap Address"=1933, "VISA Unmap Trigger"=2312, "VISA USB Control In"=2086, "VISA USB Control Out"=2087, "VISA VXI Cmd or Query"=2305, "VISA Wait On Event"=1943, "VISA Write"=1926, "VISA Write From File"=2314, "Vitesse de la lumière dans le vide (m/s)"=23518, "Vérificateur de soupape"=3833, "Wait for GPIB RQS"=1952, "WaitSRQ"=1990, "Échangeur"=3828, "Écrire dans un fichier"=1408, "Écrire dans un fichier journal LabVIEW"=8079, "Écrire plusieurs éléments dans le flux"=23804, "Écrire sur un périphérique"=1431, "Écrire sur une FIFO RT"=24002, "Écrire un seul élément dans le flux"=23798, "Écrire une variable"=23782, "Écrire une variable avec timeout"=23789, "Écriture directe de la variable "=23788, "Écriture par balayage de la variable"=23787, "Égal à 0 ?"=1113, "Égalité des nombres à virgule flottante ?"=23064, "Égaux ?"=1102, "Élément de menu sélectionné"=9001, "Élément utilisateur"=3506, "Établir une connexion à une variable"=23779, "Établir une connexion à une variable en arrière-plan"=23791, "État"=2198, "État de la fenêtre d'aide"=1354, "Étiquette libre"=2321]
          # "Creates case structure\ninside While loop"
          # "Connects init enum to shift register"
          n32 = Add(x=T3 {"Horizontal"=80, "Vertical"=-90} ("position"), y=w49) -> (x+y=w81:T1)
          n33 = New VI Object(vi object class=w107, owner refnum=w45, style=w109, position/next to=w81, 4:T2 {"Width"=300, "Height"=200} ("limites"), 8:w46) -> (object refnum=w106:refnum<vi>, 0:w80:errorcluster)  [unwired: 2 in]
          n34 = invoke class="WLoop" method="Add Shift Register"(reference=w106, error in=w80, "Y Positon"=u32 100 ("Position Y")) -> (reference out=w86:refnum<vi>, error out=w73:errorcluster, "Add Shift Register"=w104:refnum<vi>)  [unwired: 1 in, 1 out]
          n35 = property class="RShftReg"(reference=w104, error in=w73) -> (reference out=w74:refnum<vi>, error out=w72:errorcluster, "LeftRegs[]"=w103:refnum<vi>[], "InsideTerms[]"=w75:refnum<vi>[])
          n36 = property class="WLoop"(reference=w86, error in=w73) -> (reference out=w54:refnum<vi>, error out=w79:errorcluster, "LpEndRef"=w85:refnum<vi>)
          n37 = To Variant(anything=FALSE) -> (Variant=w83:variant)
          n38 = invoke class="Term" method="Create Control"(reference=w85, error in=w79, "Value"=w83) -> (reference out=w78:refnum<vi>, error out=w30:errorcluster, "Create Control"=w35:refnum<vi>)  [unwired: 1 in, 1 out]
          n39 = Index Array(array=w103) -> (element=w102:refnum<vi>)  [unwired: 1 in]
          n40 = Index Array(array=w75) -> (element=w88:refnum<vi>)  [unwired: 1 in]
          n41 = Close Reference(reference=w74, error in (no error)=w72) -> (error out=w71:errorcluster)
          n42 = property class="LShftReg"(reference=w102, error in=w71) -> (error out=w70:errorcluster, "InsideTerms[]"=w95:refnum<vi>[], "Outer Term"=w100:refnum<vi>)  [unwired: 1 out]
          n43 = property class="Ctl"(reference=w35, error in=w30, "Label.Text"="Stop") -> (reference out=w32:refnum<vi>, error out=w31:errorcluster)
          n44 = invoke class="OutrTerm" method="Connect Wire"(reference=w100, error in=w70, "Wire Source"=w47) -> (reference out=w69:refnum<vi>, error out=w68:errorcluster)  [unwired: 4 in, 5 out]
          n45 = Close Reference(reference=w32, error in (no error)=w31) -> (error out=w33:errorcluster)
          n46 = Close Reference(reference=w78, error in (no error)=w33) -> (error out=w77:errorcluster)
          n47 = Close Reference(reference=w69, error in (no error)=w68) -> (error out=w67:errorcluster)
          n48 = New VI Object(vi object class=w98, owner refnum=w54, style=w99, position/next to=T3 {"Horizontal"=20, "Vertical"=28} ("position"), 4:T2 {"Width"=220, "Height"=120} ("limites"), 8:w77) -> (object refnum=w41:refnum<vi>, 0:w76:errorcluster)  [unwired: 2 in]
          n49 = Close Reference(reference=w54, error in (no error)=w76) -> (error out=w37:errorcluster)
          n50 = property class="CaseSel"(reference=w41, error in=w37) -> (error out=w36:errorcluster, "Position"=w40:T1)  [unwired: 1 out]
          n51 = Add(x=w40, y=T1 {"Left"=0, "Top"=60} ("Sélecteur.Position")) -> (x+y=w38:T1)
          n52 = property class="CaseSel"(reference=w41, error in=w36, "Selector.Position"=w38) -> (reference out=w92:refnum<vi>, error out=w63:errorcluster, "Selector.Outer Term"=w64:refnum<vi>, "FrameCount"=w43:i32)
          n53 = Index Array(array=w95) -> (element=w94:refnum<vi>)  [unwired: 1 in]
          n54 = invoke class="InrTerm" method="Connect Wire"(reference=w94, error in=w67, "Wire Source"=w64) -> (reference out=w66:refnum<vi>, error out=w65:errorcluster)  [unwired: 4 in, 5 out]
          n55 = Decrement(x=w43) -> (x-1=w42:i32)
          n56 = Subtract(x=w48, y=u32 2) -> (x-y=w93:u32)
          n57 = Close Reference(reference=w66, error in (no error)=w65) -> (error out=w53:errorcluster)
          n58 = for {
            N: w93 -> [_]
            tunnel: w63 -> [w166]
            tunnel: [w165] -> w62
            shift-right: [w167] -> w91
            shift-left: w92 -> [w168]
            shift-right: [w163] -> _
            shift-left: w42 -> [w164]
            # "Add missing enum cases"
            n59 = invoke class="CaseSel" method="Add Frame"(reference=w168, error in=w166, "Reference Frame Index"=w164) -> (reference out=w167:refnum<vi>, error out=w165:errorcluster)  [unwired: 2 in, 3 out]
            n60 = Increment(x=w164) -> (x+1=w163:i32)
          }
          n61 = Close Reference(reference=w64, error in (no error)=w53) -> (error out=w52:errorcluster)
          n62 = Merge Errors(w46, w52) -> (w51:errorcluster)
          n63 = property class="CaseSel"(reference=w91, error in=w62) -> (reference out=w87:refnum<vi>, error out=w50:errorcluster, "Frames[]"=w89:refnum<vi>[])
          n64 = Array Size(array=w89) -> (size(s)=w90:i32)
          n65 = for "Boucle For" {
            N: w90 -> [_]
            tunnel: w89 -> [w129] mode=indexing
            tunnel: w48 -> [w126]
            tunnel: w47 -> [w123]
            tunnel: w88 -> [w119]
            tunnel: w87 -> [w118]
            tunnel: [w116] -> w61
            tunnel: [w115] -> w59
            tunnel: [w112] -> w57
            tunnel: [w111] -> w56
            tunnel: w50 -> [w110]
            i -> [w117]
            # "Duplicates enum and inserts a single instance into each case + wires all the enums"
            n66 = Increment(x=w117) -> (x+1=w128:i32)
            n67 = Quotient & Remainder(x=w128, y=w126) -> (x-y*floor(x/y)=w127:u32)  [unwired: 1 out]
            n68 = To Variant(anything=w127) -> (Variant=w124:variant)
            n69 = invoke class="Term" method="Create Constant"(reference=w123, error in=w110, "Value"=w124) -> (reference out=w112:refnum<vi>, error out=w113:errorcluster, "Create Constant"=w122:refnum<vi>)  [unwired: 1 in, 1 out]
            n70 = invoke class="Const" method="Move"(reference=w122, error in=w113, "position"=T1 {"Left"=100, "Top"=50}, "owner"=w129, "duplicate"=FALSE ("Dupliquer ? (F)")) -> (reference out=w120:refnum<vi>, error out=w114:errorcluster)  [unwired: 1 in, 4 out]
            n71 = case shown="1, 默认" w117 {
              selector: w117 -> [w145 _]
              tunnel: w120 -> [w146 w162]
              tunnel: w119 -> [w144 w161]
              tunnel: w118 -> [w150 w159]
              tunnel: [w144 w160] -> w116
              tunnel: [w135 w159] -> w115
              tunnel: w114 -> [w130 w153]
              tunnel: [w133 w152] -> w111
              frame 1, Default {
                n72 = property class="CaseSel"(reference=w150, error in=w130) -> (reference out=w135:refnum<vi>, error out=w139:errorcluster, "Tunnels[]"=w151:refnum<vi>[])
                n73 = Index Array(array=w151) -> (element=w149:refnum<vi>)  [unwired: 1 in]
                n74 = property class="Tun"(reference=w149, error in=w139) -> (reference out=w138:refnum<vi>, error out=w140:errorcluster, "InsideTerms[]"=w148:refnum<vi>[])
                n75 = property class="Const"(reference=w146, error in=w140) -> (reference out=w136:refnum<vi>, error out=w141:errorcluster, "Terminal"=w137:refnum<vi>)
                n76 = Index Array(array=w148, index=w145) -> (element=w147:refnum<vi>)
                n77 = invoke class="InrTerm" method="Connect Wire"(reference=w147, error in=w141, "Wire Source"=w137) -> (reference out=w143:refnum<vi>, error out=w142:errorcluster)  [unwired: 4 in, 5 out]
                n78 = Close Reference(reference=w143, error in (no error)=w142) -> (error out=w131:errorcluster)
                n79 = Close Reference(reference=w137, error in (no error)=w131) -> (error out=w132:errorcluster)
                n80 = Close Reference(reference=w136, error in (no error)=w132) -> (error out=w134:errorcluster)
                n81 = Close Reference(reference=w138, error in (no error)=w134) -> (error out=w133:errorcluster)
              }
              frame 0 {
                n82 = property class="Const"(reference=w162, error in=w153) -> (reference out=w156:refnum<vi>, error out=w154:errorcluster, "Terminal"=w158:refnum<vi>)
                n83 = invoke class="InrTerm" method="Connect Wire"(reference=w161, error in=w154, "Wire Source"=w158) -> (reference out=w160:refnum<vi>, error out=w155:errorcluster)  [unwired: 4 in, 5 out]
                n84 = Close Reference(reference=w158, error in (no error)=w155) -> (error out=w157:errorcluster)
                n85 = Close Reference(reference=w156, error in (no error)=w157) -> (error out=w152:errorcluster)
              }
            }
          }
          n86 = Close Reference(reference=w61, error in (no error)=w56) -> (error out=w60:errorcluster)
          n87 = Close Reference(reference=w59, error in (no error)=w60) -> (error out=w58:errorcluster)
          n88 = Close Reference(reference=w57, error in (no error)=w58) -> (error out=w55:errorcluster)
          n89 = Merge Errors(w51, w55) -> (w44:errorcluster)
        }
        frame Error {
        }
      }
      n90 = invoke class="VI" method="Transaction.End Undo"(reference=w9, error in=w13) -> (error out=w23:errorcluster)  [unwired: 1 in, 2 out]
    }
    frame Error {
    }
  }
  "error out" <- w7
  "Variant out" <- w1
